vi "Tausand AB1000 Acquisition Example.vi"() -> ()   [LabVIEW 2015]
doc: "Example of a complete acquisition system using a Tausand Abacus.\n\nIncludes device identification, live settings changes and live data reading.\nData is shown in tables, graphs and saved in plain text files.\nUses a producer-consumer design pattern."
uses:
  <instrlib>/Tausand AB1000/Examples/sub vi/connectionState.ctl
  <instrlib>/Tausand AB1000/Public/Controls/settings4ch.ctl
  <instrlib>/Tausand AB1000/Public/Controls/configMultipleCoincRing.ctl
  <instrlib>/Tausand AB1000/Examples/sub vi/defaultSettings.ctl
  <instrlib>/Tausand AB1000/Public/Controls/deviceTypeRing.ctl
  <instrlib>/Tausand AB1000/Public/Controls/settings2ch.ctl
  <instrlib>/Tausand AB1000/Public/Controls/counters2ch.ctl
  <instrlib>/Tausand AB1000/Public/Controls/counters4ch.ctl
  <vilib>/Utility/miscctls.llb/LVRowAndColumnUnsignedTypeDef.ctl
  <instrlib>/Tausand AB1000/Public/Controls/channelRing.ctl
  <vilib>/Utility/file.llb/Write Delimited Spreadsheet (string).vi
  <vilib>/Utility/file.llb/Read Delimited Spreadsheet (string).vi
  <instrlib>/Tausand AB1000/Tausand AB1000.lvlib
panel:
  out "ref ctrls":T1
  out "timer-settings 2":timestamp
  in  "butLoadDefSett":bool
  out "ref indics":T2
  out "dafafile header":string[](array[string])
  in  "settings 2ch":T3={"sampling"=1000, "coincidence_window"=10, "delay_A"=0, "delay_B"=0, "sleep_A"=0, "sleep_B"=0} {"sleep_B" max=100 step=5; "sleep_A" max=100 step=5; "delay_B" max=100 step=5; "delay_A" max=100 step=5; "coincidence_window" min=5 max=50000 step=5; "sampling" items=["1ms"=1, "2ms"=2, "5ms"=5, "10ms"=10, "20ms"=20, "50ms"=50, "100ms"=100, "200ms"=200, "500ms"=500, "1s"=1000, "2s"=2000, "5s"=5000, "10s"=10000, "20s"=20000, "50s"=50000, "100s"=100000, "200s"=200000, "500s"=500000, "1000s"=1000000]}
  in  "settings 4ch":T4={"sampling"=1000, "coincidence_window"=10, "delay_A"=0, "delay_B"=0, "delay_C"=0, "delay_D"=0, "sleep_A"=0, "sleep_B"=0, "sleep_C"=0, "sleep_D"=0, "config_multiple_1"=240} {"config_multiple_1" items=["ABC"=224, "ABD"=208, "ACD"=176, "BCD"=112, "ABCD"=240]; "sleep_D" max=100 step=5; "sleep_C" max=100 step=5; "sleep_B" max=100 step=5; "sleep_A" max=100 step=5; "delay_D" max=100 step=5; "delay_C" max=100 step=5; "delay_B" max=100 step=5; "delay_A" max=100 step=5; "coincidence_window" min=5 max=10000 step=5; "sampling" items=["1ms"=1, "2ms"=2, "3ms"=3, "4ms"=4, "5ms"=5, "6ms"=6, "7ms"=7, "8ms"=8, "9ms"=9, "10ms"=10, "11ms"=11, "12ms"=12, "13ms"=13, "14ms"=14, "15ms"=15, "16ms"=16, "17ms"=17, "18ms"=18, "19ms"=19, "20ms"=20, "21ms"=21, "22ms"=22, "23ms"=23, "24ms"=24, "25ms"=25, "26ms"=26, "27ms"=27, "28ms"=28, "29ms"=29, "30ms"=30, "31ms"=31, "32ms"=32, "33ms"=33, "34ms"=34, "35ms"=35, "36ms"=36, "37ms"=37, "38ms"=38, "39ms"=39, "40ms"=40, "41ms"=41, "42ms"=42, "43ms"=43, "44ms"=44, "45ms"=45, "46ms"=46, "47ms"=47, "48ms"=48, "49ms"=49, "50ms"=50, "51ms"=51, "52ms"=52, "53ms"=53, "54ms"=54, "55ms"=55, "56ms"=56, "57ms"=57, "58ms"=58, "59ms"=59, "60ms"=60, "61ms"=61, "62ms"=62, "63ms"=63, "64ms"=64, "65ms"=65, "66ms"=66, "67ms"=67, "68ms"=68, "69ms"=69, "70ms"=70, "71ms"=71, "72ms"=72, "73ms"=73, "74ms"=74, "75ms"=75, "76ms"=76, "77ms"=77, "78ms"=78, "79ms"=79, "80ms"=80, "81ms"=81, "82ms"=82, "83ms"=83, "84ms"=84, "85ms"=85, "86ms"=86, "87ms"=87, "88ms"=88, "89ms"=89, "90ms"=90, "91ms"=91, "92ms"=92, "93ms"=93, "94ms"=94, "95ms"=95, "96ms"=96, "97ms"=97, "98ms"=98, "99ms"=99, "100ms"=100, "110ms"=110, "120ms"=120, "130ms"=130, "140ms"=140, "150ms"=150, "160ms"=160, "170ms"=170, "180ms"=180, "190ms"=190, "200ms"=200, "210ms"=210, "220ms"=220, "230ms"=230, "240ms"=240, "250ms"=250, "260ms"=260, "270ms"=270, "280ms"=280, "290ms"=290, "300ms"=300, "310ms"=310, "320ms"=320, "330ms"=330, "340ms"=340, "350ms"=350, "360ms"=360, "370ms"=370, "380ms"=380, "390ms"=390, "400ms"=400, "410ms"=410, "420ms"=420, "430ms"=430, "440ms"=440, "450ms"=450, "460ms"=460, "470ms"=470, "480ms"=480, "490ms"=490, "500ms"=500, "510ms"=510, "520ms"=520, "530ms"=530, "540ms"=540, "550ms"=550, "560ms"=560, "570ms"=570, "580ms"=580, "590ms"=590, "600ms"=600, "610ms"=610, "620ms"=620, "630ms"=630, "640ms"=640, "650ms"=650, "660ms"=660, "670ms"=670, "680ms"=680, "690ms"=690, "700ms"=700, "710ms"=710, "720ms"=720, "730ms"=730, "740ms"=740, "750ms"=750, "760ms"=760, "770ms"=770, "780ms"=780, "790ms"=790, "800ms"=800, "810ms"=810, "820ms"=820, "830ms"=830, "840ms"=840, "850ms"=850, "860ms"=860, "870ms"=870, "880ms"=880, "890ms"=890, "900ms"=900, "910ms"=910, "920ms"=920, "930ms"=930, "940ms"=940, "950ms"=950, "960ms"=960, "970ms"=970, "980ms"=980, "990ms"=990, "1,0s"=1000, "1,1s"=1100, "1,2s"=1200, "1,3s"=1300, "1,4s"=1400, "1,5s"=1500, "1,6s"=1600, "1,7s"=1700, "1,8s"=1800, "1,9s"=1900, "2,0s"=2000, "2,1s"=2100, "2,2s"=2200, "2,3s"=2300, "2,4s"=2400, "2,5s"=2500, "2,6s"=2600, "2,7s"=2700, "2,8s"=2800, "2,9s"=2900, "3,0s"=3000, "3,1s"=3100, "3,2s"=3200, "3,3s"=3300, "3,4s"=3400, "3,5s"=3500, "3,6s"=3600, "3,7s"=3700, "3,8s"=3800, "3,9s"=3900, "4,0s"=4000, "4,1s"=4100, "4,2s"=4200, "4,3s"=4300, "4,4s"=4400, "4,5s"=4500, "4,6s"=4600, "4,7s"=4700, "4,8s"=4800, "4,9s"=4900, "5,0s"=5000, "5,1s"=5100, "5,2s"=5200, "5,3s"=5300, "5,4s"=5400, "5,5s"=5500, "5,6s"=5600, "5,7s"=5700, "5,8s"=5800, "5,9s"=5900, "6,0s"=6000, "6,1s"=6100, "6,2s"=6200, "6,3s"=6300, "6,4s"=6400, "6,5s"=6500, "6,6s"=6600, "6,7s"=6700, "6,8s"=6800, "6,9s"=6900, "7,0s"=7000, "7,1s"=7100, "7,2s"=7200, "7,3s"=7300, "7,4s"=7400, "7,5s"=7500, "7,6s"=7600, "7,7s"=7700, "7,8s"=7800, "7,9s"=7900, "8,0s"=8000, "8,1s"=8100, "8,2s"=8200, "8,3s"=8300, "8,4s"=8400, "8,5s"=8500, "8,6s"=8600, "8,7s"=8700, "8,8s"=8800, "8,9s"=8900, "9,0s"=9000, "9,1s"=9100, "9,2s"=9200, "9,3s"=9300, "9,4s"=9400, "9,5s"=9500, "9,6s"=9600, "9,7s"=9700, "9,8s"=9800, "9,9s"=9900, "10s"=10000, "11s"=11000, "12s"=12000, "13s"=13000, "14s"=14000, "15s"=15000, "16s"=16000, "17s"=17000, "18s"=18000, "19s"=19000, "20s"=20000, "21s"=21000, "22s"=22000, "23s"=23000, "24s"=24000, "25s"=25000, "26s"=26000, "27s"=27000, "28s"=28000, "29s"=29000, "30s"=30000, "31s"=31000, "32s"=32000, "33s"=33000, "34s"=34000, "35s"=35000, "36s"=36000, "37s"=37000, "38s"=38000, "39s"=39000, "40s"=40000, "41s"=41000, "42s"=42000, "43s"=43000, "44s"=44000, "45s"=45000, "46s"=46000, "47s"=47000, "48s"=48000, "49s"=49000, "50s"=50000, "51s"=51000, "52s"=52000, "53s"=53000, "54s"=54000, "55s"=55000, "56s"=56000, "57s"=57000, "58s"=58000, "59s"=59000, "60s"=60000, "61s"=61000, "62s"=62000, "63s"=63000, "64s"=64000, "65s"=65000, "66s"=66000, "67s"=67000, "68s"=68000, "69s"=69000, "70s"=70000, "71s"=71000, "72s"=72000, "73s"=73000, "74s"=74000, "75s"=75000, "76s"=76000, "77s"=77000, "78s"=78000, "79s"=79000, "80s"=80000, "81s"=81000, "82s"=82000, "83s"=83000, "84s"=84000, "85s"=85000, "86s"=86000, "87s"=87000, "88s"=88000, "89s"=89000, "90s"=90000, "91s"=91000, "92s"=92000, "93s"=93000, "94s"=94000, "95s"=95000, "96s"=96000, "97s"=97000, "98s"=98000, "99s"=99000, "100s"=100000, "110s"=110000, "120s"=120000, "130s"=130000, "140s"=140000, "150s"=150000, "160s"=160000, "170s"=170000, "180s"=180000, "190s"=190000, "200s"=200000, "210s"=210000, "220s"=220000, "230s"=230000, "240s"=240000, "250s"=250000, "260s"=260000, "270s"=270000, "280s"=280000, "290s"=290000, "300s"=300000, "310s"=310000, "320s"=320000, "330s"=330000, "340s"=340000, "350s"=350000, "360s"=360000, "370s"=370000, "380s"=380000, "390s"=390000, "400s"=400000, "410s"=410000, "420s"=420000, "430s"=430000, "440s"=440000, "450s"=450000, "460s"=460000, "470s"=470000, "480s"=480000, "490s"=490000, "500s"=500000, "510s"=510000, "520s"=520000, "530s"=530000, "540s"=540000, "550s"=550000, "560s"=560000, "570s"=570000, "580s"=580000, "590s"=590000, "600s"=600000, "610s"=610000, "620s"=620000, "630s"=630000, "640s"=640000, "650s"=650000, "660s"=660000, "670s"=670000, "680s"=680000, "690s"=690000, "700s"=700000, "710s"=710000, "720s"=720000, "730s"=730000, "740s"=740000, "750s"=750000, "760s"=760000, "770s"=770000, "780s"=780000, "790s"=790000, "800s"=800000, "810s"=810000, "820s"=820000, "830s"=830000, "840s"=840000, "850s"=850000, "860s"=860000, "870s"=870000, "880s"=880000, "890s"=890000, "900s"=900000, "910s"=910000, "920s"=920000, "930s"=930000, "940s"=940000, "950s"=950000, "960s"=960000, "970s"=970000, "980s"=980000, "990s"=990000, "1000s"=1000000]}
  out "device type":T6 items=["any"=0, "AB1002"=1002, "AB1004"=1004, "AB1502"=1502, "AB1504"=1504, "AB2002"=2002, "AB2004"=2004, "AB2502"=2502, "AB2504"=2504]
  out "path-defsettings":path
  out "delimiter":string
  out "default settings":T7={"autogenerate"=FALSE, "datetime"=FALSE, "from_device"=FALSE, "directory"="", "file_prefix"="", "settings_suffix"="", "delimiter"="", "extension"="", "Abacus settings"={"sampling"=0, "coincidence_window"=0, "delay_A"=0, "delay_B"=0, "delay_C"=0, "delay_D"=0, "sleep_A"=0, "sleep_B"=0, "sleep_C"=0, "sleep_D"=0, "config_multiple_1"=240}} {"Abacus settings"."config_multiple_1" items=["ABC"=224, "ABD"=208, "ACD"=176, "BCD"=112, "ABCD"=240]; "Abacus settings"."sleep_D" max=100 step=5; "Abacus settings"."sleep_C" max=100 step=5; "Abacus settings"."sleep_B" max=100 step=5; "Abacus settings"."sleep_A" max=100 step=5; "Abacus settings"."delay_D" max=100 step=5; "Abacus settings"."delay_C" max=100 step=5; "Abacus settings"."delay_B" max=100 step=5; "Abacus settings"."delay_A" max=100 step=5; "Abacus settings"."coincidence_window" min=5 max=10000 step=5; "Abacus settings"."sampling" items=["1ms"=1, "2ms"=2, "3ms"=3, "4ms"=4, "5ms"=5, "6ms"=6, "7ms"=7, "8ms"=8, "9ms"=9, "10ms"=10, "11ms"=11, "12ms"=12, "13ms"=13, "14ms"=14, "15ms"=15, "16ms"=16, "17ms"=17, "18ms"=18, "19ms"=19, "20ms"=20, "21ms"=21, "22ms"=22, "23ms"=23, "24ms"=24, "25ms"=25, "26ms"=26, "27ms"=27, "28ms"=28, "29ms"=29, "30ms"=30, "31ms"=31, "32ms"=32, "33ms"=33, "34ms"=34, "35ms"=35, "36ms"=36, "37ms"=37, "38ms"=38, "39ms"=39, "40ms"=40, "41ms"=41, "42ms"=42, "43ms"=43, "44ms"=44, "45ms"=45, "46ms"=46, "47ms"=47, "48ms"=48, "49ms"=49, "50ms"=50, "51ms"=51, "52ms"=52, "53ms"=53, "54ms"=54, "55ms"=55, "56ms"=56, "57ms"=57, "58ms"=58, "59ms"=59, "60ms"=60, "61ms"=61, "62ms"=62, "63ms"=63, "64ms"=64, "65ms"=65, "66ms"=66, "67ms"=67, "68ms"=68, "69ms"=69, "70ms"=70, "71ms"=71, "72ms"=72, "73ms"=73, "74ms"=74, "75ms"=75, "76ms"=76, "77ms"=77, "78ms"=78, "79ms"=79, "80ms"=80, "81ms"=81, "82ms"=82, "83ms"=83, "84ms"=84, "85ms"=85, "86ms"=86, "87ms"=87, "88ms"=88, "89ms"=89, "90ms"=90, "91ms"=91, "92ms"=92, "93ms"=93, "94ms"=94, "95ms"=95, "96ms"=96, "97ms"=97, "98ms"=98, "99ms"=99, "100ms"=100, "110ms"=110, "120ms"=120, "130ms"=130, "140ms"=140, "150ms"=150, "160ms"=160, "170ms"=170, "180ms"=180, "190ms"=190, "200ms"=200, "210ms"=210, "220ms"=220, "230ms"=230, "240ms"=240, "250ms"=250, "260ms"=260, "270ms"=270, "280ms"=280, "290ms"=290, "300ms"=300, "310ms"=310, "320ms"=320, "330ms"=330, "340ms"=340, "350ms"=350, "360ms"=360, "370ms"=370, "380ms"=380, "390ms"=390, "400ms"=400, "410ms"=410, "420ms"=420, "430ms"=430, "440ms"=440, "450ms"=450, "460ms"=460, "470ms"=470, "480ms"=480, "490ms"=490, "500ms"=500, "510ms"=510, "520ms"=520, "530ms"=530, "540ms"=540, "550ms"=550, "560ms"=560, "570ms"=570, "580ms"=580, "590ms"=590, "600ms"=600, "610ms"=610, "620ms"=620, "630ms"=630, "640ms"=640, "650ms"=650, "660ms"=660, "670ms"=670, "680ms"=680, "690ms"=690, "700ms"=700, "710ms"=710, "720ms"=720, "730ms"=730, "740ms"=740, "750ms"=750, "760ms"=760, "770ms"=770, "780ms"=780, "790ms"=790, "800ms"=800, "810ms"=810, "820ms"=820, "830ms"=830, "840ms"=840, "850ms"=850, "860ms"=860, "870ms"=870, "880ms"=880, "890ms"=890, "900ms"=900, "910ms"=910, "920ms"=920, "930ms"=930, "940ms"=940, "950ms"=950, "960ms"=960, "970ms"=970, "980ms"=980, "990ms"=990, "1,0s"=1000, "1,1s"=1100, "1,2s"=1200, "1,3s"=1300, "1,4s"=1400, "1,5s"=1500, "1,6s"=1600, "1,7s"=1700, "1,8s"=1800, "1,9s"=1900, "2,0s"=2000, "2,1s"=2100, "2,2s"=2200, "2,3s"=2300, "2,4s"=2400, "2,5s"=2500, "2,6s"=2600, "2,7s"=2700, "2,8s"=2800, "2,9s"=2900, "3,0s"=3000, "3,1s"=3100, "3,2s"=3200, "3,3s"=3300, "3,4s"=3400, "3,5s"=3500, "3,6s"=3600, "3,7s"=3700, "3,8s"=3800, "3,9s"=3900, "4,0s"=4000, "4,1s"=4100, "4,2s"=4200, "4,3s"=4300, "4,4s"=4400, "4,5s"=4500, "4,6s"=4600, "4,7s"=4700, "4,8s"=4800, "4,9s"=4900, "5,0s"=5000, "5,1s"=5100, "5,2s"=5200, "5,3s"=5300, "5,4s"=5400, "5,5s"=5500, "5,6s"=5600, "5,7s"=5700, "5,8s"=5800, "5,9s"=5900, "6,0s"=6000, "6,1s"=6100, "6,2s"=6200, "6,3s"=6300, "6,4s"=6400, "6,5s"=6500, "6,6s"=6600, "6,7s"=6700, "6,8s"=6800, "6,9s"=6900, "7,0s"=7000, "7,1s"=7100, "7,2s"=7200, "7,3s"=7300, "7,4s"=7400, "7,5s"=7500, "7,6s"=7600, "7,7s"=7700, "7,8s"=7800, "7,9s"=7900, "8,0s"=8000, "8,1s"=8100, "8,2s"=8200, "8,3s"=8300, "8,4s"=8400, "8,5s"=8500, "8,6s"=8600, "8,7s"=8700, "8,8s"=8800, "8,9s"=8900, "9,0s"=9000, "9,1s"=9100, "9,2s"=9200, "9,3s"=9300, "9,4s"=9400, "9,5s"=9500, "9,6s"=9600, "9,7s"=9700, "9,8s"=9800, "9,9s"=9900, "10s"=10000, "11s"=11000, "12s"=12000, "13s"=13000, "14s"=14000, "15s"=15000, "16s"=16000, "17s"=17000, "18s"=18000, "19s"=19000, "20s"=20000, "21s"=21000, "22s"=22000, "23s"=23000, "24s"=24000, "25s"=25000, "26s"=26000, "27s"=27000, "28s"=28000, "29s"=29000, "30s"=30000, "31s"=31000, "32s"=32000, "33s"=33000, "34s"=34000, "35s"=35000, "36s"=36000, "37s"=37000, "38s"=38000, "39s"=39000, "40s"=40000, "41s"=41000, "42s"=42000, "43s"=43000, "44s"=44000, "45s"=45000, "46s"=46000, "47s"=47000, "48s"=48000, "49s"=49000, "50s"=50000, "51s"=51000, "52s"=52000, "53s"=53000, "54s"=54000, "55s"=55000, "56s"=56000, "57s"=57000, "58s"=58000, "59s"=59000, "60s"=60000, "61s"=61000, "62s"=62000, "63s"=63000, "64s"=64000, "65s"=65000, "66s"=66000, "67s"=67000, "68s"=68000, "69s"=69000, "70s"=70000, "71s"=71000, "72s"=72000, "73s"=73000, "74s"=74000, "75s"=75000, "76s"=76000, "77s"=77000, "78s"=78000, "79s"=79000, "80s"=80000, "81s"=81000, "82s"=82000, "83s"=83000, "84s"=84000, "85s"=85000, "86s"=86000, "87s"=87000, "88s"=88000, "89s"=89000, "90s"=90000, "91s"=91000, "92s"=92000, "93s"=93000, "94s"=94000, "95s"=95000, "96s"=96000, "97s"=97000, "98s"=98000, "99s"=99000, "100s"=100000, "110s"=110000, "120s"=120000, "130s"=130000, "140s"=140000, "150s"=150000, "160s"=160000, "170s"=170000, "180s"=180000, "190s"=190000, "200s"=200000, "210s"=210000, "220s"=220000, "230s"=230000, "240s"=240000, "250s"=250000, "260s"=260000, "270s"=270000, "280s"=280000, "290s"=290000, "300s"=300000, "310s"=310000, "320s"=320000, "330s"=330000, "340s"=340000, "350s"=350000, "360s"=360000, "370s"=370000, "380s"=380000, "390s"=390000, "400s"=400000, "410s"=410000, "420s"=420000, "430s"=430000, "440s"=440000, "450s"=450000, "460s"=460000, "470s"=470000, "480s"=480000, "490s"=490000, "500s"=500000, "510s"=510000, "520s"=520000, "530s"=530000, "540s"=540000, "550s"=550000, "560s"=560000, "570s"=570000, "580s"=580000, "590s"=590000, "600s"=600000, "610s"=610000, "620s"=620000, "630s"=630000, "640s"=640000, "650s"=650000, "660s"=660000, "670s"=670000, "680s"=680000, "690s"=690000, "700s"=700000, "710s"=710000, "720s"=720000, "730s"=730000, "740s"=740000, "750s"=750000, "760s"=760000, "770s"=770000, "780s"=780000, "790s"=790000, "800s"=800000, "810s"=810000, "820s"=820000, "830s"=830000, "840s"=840000, "850s"=850000, "860s"=860000, "870s"=870000, "880s"=880000, "890s"=890000, "900s"=900000, "910s"=910000, "920s"=920000, "930s"=930000, "940s"=940000, "950s"=950000, "960s"=960000, "970s"=970000, "980s"=980000, "990s"=990000, "1000s"=1000000]}
  out "settings_old":T4={"sampling"=1000, "coincidence_window"=10, "delay_A"=0, "delay_B"=0, "delay_C"=0, "delay_D"=0, "sleep_A"=0, "sleep_B"=0, "sleep_C"=0, "sleep_D"=0, "config_multiple_1"=0} {"config_multiple_1" items=["ABC"=224, "ABD"=208, "ACD"=176, "BCD"=112, "ABCD"=240]; "sleep_D" max=100 step=1; "sleep_C" max=100 step=1; "sleep_B" max=100 step=1; "sleep_A" max=100 step=1; "delay_D" max=100 step=1; "delay_C" max=100 step=1; "delay_B" max=100 step=1; "delay_A" max=100 step=1; "coincidence_window" min=1 max=10000 step=1; "sampling" items=["1ms"=1, "2ms"=2, "3ms"=3, "4ms"=4, "5ms"=5, "6ms"=6, "7ms"=7, "8ms"=8, "9ms"=9, "10ms"=10, "11ms"=11, "12ms"=12, "13ms"=13, "14ms"=14, "15ms"=15, "16ms"=16, "17ms"=17, "18ms"=18, "19ms"=19, "20ms"=20, "21ms"=21, "22ms"=22, "23ms"=23, "24ms"=24, "25ms"=25, "26ms"=26, "27ms"=27, "28ms"=28, "29ms"=29, "30ms"=30, "31ms"=31, "32ms"=32, "33ms"=33, "34ms"=34, "35ms"=35, "36ms"=36, "37ms"=37, "38ms"=38, "39ms"=39, "40ms"=40, "41ms"=41, "42ms"=42, "43ms"=43, "44ms"=44, "45ms"=45, "46ms"=46, "47ms"=47, "48ms"=48, "49ms"=49, "50ms"=50, "51ms"=51, "52ms"=52, "53ms"=53, "54ms"=54, "55ms"=55, "56ms"=56, "57ms"=57, "58ms"=58, "59ms"=59, "60ms"=60, "61ms"=61, "62ms"=62, "63ms"=63, "64ms"=64, "65ms"=65, "66ms"=66, "67ms"=67, "68ms"=68, "69ms"=69, "70ms"=70, "71ms"=71, "72ms"=72, "73ms"=73, "74ms"=74, "75ms"=75, "76ms"=76, "77ms"=77, "78ms"=78, "79ms"=79, "80ms"=80, "81ms"=81, "82ms"=82, "83ms"=83, "84ms"=84, "85ms"=85, "86ms"=86, "87ms"=87, "88ms"=88, "89ms"=89, "90ms"=90, "91ms"=91, "92ms"=92, "93ms"=93, "94ms"=94, "95ms"=95, "96ms"=96, "97ms"=97, "98ms"=98, "99ms"=99, "100ms"=100, "110ms"=110, "120ms"=120, "130ms"=130, "140ms"=140, "150ms"=150, "160ms"=160, "170ms"=170, "180ms"=180, "190ms"=190, "200ms"=200, "210ms"=210, "220ms"=220, "230ms"=230, "240ms"=240, "250ms"=250, "260ms"=260, "270ms"=270, "280ms"=280, "290ms"=290, "300ms"=300, "310ms"=310, "320ms"=320, "330ms"=330, "340ms"=340, "350ms"=350, "360ms"=360, "370ms"=370, "380ms"=380, "390ms"=390, "400ms"=400, "410ms"=410, "420ms"=420, "430ms"=430, "440ms"=440, "450ms"=450, "460ms"=460, "470ms"=470, "480ms"=480, "490ms"=490, "500ms"=500, "510ms"=510, "520ms"=520, "530ms"=530, "540ms"=540, "550ms"=550, "560ms"=560, "570ms"=570, "580ms"=580, "590ms"=590, "600ms"=600, "610ms"=610, "620ms"=620, "630ms"=630, "640ms"=640, "650ms"=650, "660ms"=660, "670ms"=670, "680ms"=680, "690ms"=690, "700ms"=700, "710ms"=710, "720ms"=720, "730ms"=730, "740ms"=740, "750ms"=750, "760ms"=760, "770ms"=770, "780ms"=780, "790ms"=790, "800ms"=800, "810ms"=810, "820ms"=820, "830ms"=830, "840ms"=840, "850ms"=850, "860ms"=860, "870ms"=870, "880ms"=880, "890ms"=890, "900ms"=900, "910ms"=910, "920ms"=920, "930ms"=930, "940ms"=940, "950ms"=950, "960ms"=960, "970ms"=970, "980ms"=980, "990ms"=990, "1,0s"=1000, "1,1s"=1100, "1,2s"=1200, "1,3s"=1300, "1,4s"=1400, "1,5s"=1500, "1,6s"=1600, "1,7s"=1700, "1,8s"=1800, "1,9s"=1900, "2,0s"=2000, "2,1s"=2100, "2,2s"=2200, "2,3s"=2300, "2,4s"=2400, "2,5s"=2500, "2,6s"=2600, "2,7s"=2700, "2,8s"=2800, "2,9s"=2900, "3,0s"=3000, "3,1s"=3100, "3,2s"=3200, "3,3s"=3300, "3,4s"=3400, "3,5s"=3500, "3,6s"=3600, "3,7s"=3700, "3,8s"=3800, "3,9s"=3900, "4,0s"=4000, "4,1s"=4100, "4,2s"=4200, "4,3s"=4300, "4,4s"=4400, "4,5s"=4500, "4,6s"=4600, "4,7s"=4700, "4,8s"=4800, "4,9s"=4900, "5,0s"=5000, "5,1s"=5100, "5,2s"=5200, "5,3s"=5300, "5,4s"=5400, "5,5s"=5500, "5,6s"=5600, "5,7s"=5700, "5,8s"=5800, "5,9s"=5900, "6,0s"=6000, "6,1s"=6100, "6,2s"=6200, "6,3s"=6300, "6,4s"=6400, "6,5s"=6500, "6,6s"=6600, "6,7s"=6700, "6,8s"=6800, "6,9s"=6900, "7,0s"=7000, "7,1s"=7100, "7,2s"=7200, "7,3s"=7300, "7,4s"=7400, "7,5s"=7500, "7,6s"=7600, "7,7s"=7700, "7,8s"=7800, "7,9s"=7900, "8,0s"=8000, "8,1s"=8100, "8,2s"=8200, "8,3s"=8300, "8,4s"=8400, "8,5s"=8500, "8,6s"=8600, "8,7s"=8700, "8,8s"=8800, "8,9s"=8900, "9,0s"=9000, "9,1s"=9100, "9,2s"=9200, "9,3s"=9300, "9,4s"=9400, "9,5s"=9500, "9,6s"=9600, "9,7s"=9700, "9,8s"=9800, "9,9s"=9900, "10s"=10000, "11s"=11000, "12s"=12000, "13s"=13000, "14s"=14000, "15s"=15000, "16s"=16000, "17s"=17000, "18s"=18000, "19s"=19000, "20s"=20000, "21s"=21000, "22s"=22000, "23s"=23000, "24s"=24000, "25s"=25000, "26s"=26000, "27s"=27000, "28s"=28000, "29s"=29000, "30s"=30000, "31s"=31000, "32s"=32000, "33s"=33000, "34s"=34000, "35s"=35000, "36s"=36000, "37s"=37000, "38s"=38000, "39s"=39000, "40s"=40000, "41s"=41000, "42s"=42000, "43s"=43000, "44s"=44000, "45s"=45000, "46s"=46000, "47s"=47000, "48s"=48000, "49s"=49000, "50s"=50000, "51s"=51000, "52s"=52000, "53s"=53000, "54s"=54000, "55s"=55000, "56s"=56000, "57s"=57000, "58s"=58000, "59s"=59000, "60s"=60000, "61s"=61000, "62s"=62000, "63s"=63000, "64s"=64000, "65s"=65000, "66s"=66000, "67s"=67000, "68s"=68000, "69s"=69000, "70s"=70000, "71s"=71000, "72s"=72000, "73s"=73000, "74s"=74000, "75s"=75000, "76s"=76000, "77s"=77000, "78s"=78000, "79s"=79000, "80s"=80000, "81s"=81000, "82s"=82000, "83s"=83000, "84s"=84000, "85s"=85000, "86s"=86000, "87s"=87000, "88s"=88000, "89s"=89000, "90s"=90000, "91s"=91000, "92s"=92000, "93s"=93000, "94s"=94000, "95s"=95000, "96s"=96000, "97s"=97000, "98s"=98000, "99s"=99000, "100s"=100000, "110s"=110000, "120s"=120000, "130s"=130000, "140s"=140000, "150s"=150000, "160s"=160000, "170s"=170000, "180s"=180000, "190s"=190000, "200s"=200000, "210s"=210000, "220s"=220000, "230s"=230000, "240s"=240000, "250s"=250000, "260s"=260000, "270s"=270000, "280s"=280000, "290s"=290000, "300s"=300000, "310s"=310000, "320s"=320000, "330s"=330000, "340s"=340000, "350s"=350000, "360s"=360000, "370s"=370000, "380s"=380000, "390s"=390000, "400s"=400000, "410s"=410000, "420s"=420000, "430s"=430000, "440s"=440000, "450s"=450000, "460s"=460000, "470s"=470000, "480s"=480000, "490s"=490000, "500s"=500000, "510s"=510000, "520s"=520000, "530s"=530000, "540s"=540000, "550s"=550000, "560s"=560000, "570s"=570000, "580s"=580000, "590s"=590000, "600s"=600000, "610s"=610000, "620s"=620000, "630s"=630000, "640s"=640000, "650s"=650000, "660s"=660000, "670s"=670000, "680s"=680000, "690s"=690000, "700s"=700000, "710s"=710000, "720s"=720000, "730s"=730000, "740s"=740000, "750s"=750000, "760s"=760000, "770s"=770000, "780s"=780000, "790s"=790000, "800s"=800000, "810s"=810000, "820s"=820000, "830s"=830000, "840s"=840000, "850s"=850000, "860s"=860000, "870s"=870000, "880s"=880000, "890s"=890000, "900s"=900000, "910s"=910000, "920s"=920000, "930s"=930000, "940s"=940000, "950s"=950000, "960s"=960000, "970s"=970000, "980s"=980000, "990s"=990000, "1000s"=1000000]}
  out "sttgs changed?":bool[](array[boolean])
  out "connection state":T8
  out "timer-reconnect":timestamp
  out "status":string
  out "path-new":path
  out "error":errorcluster
  out "path-settingsOld":path
  out "path-settings":path
  out "timer-settings":timestamp
  out "timer-readRequest":timestamp
  in  "Tab Control":T9(tab)
  out "dataTable":string[][](table)
  out "counters 2ch":T10
  out "counters 4ch":T11
  out "graph-A":cluster{timestamp[], u32[]}(graph) caption="small graph A"
  out "graph-B":cluster{timestamp[], u32[]}(graph) caption="small graph B"
  out "graph-C":cluster{timestamp[], u32[]}(graph) caption="small graph C"
  out "graph-D":cluster{timestamp[], u32[]}(graph) caption="small graph D"
  out "graph coinc":cluster{timestamp[], u32[]}[](graph)
  out "graph-A-S":cluster{timestamp[], u32[]}(graph) caption="small graph A"
  out "graph-B-S":cluster{timestamp[], u32[]}(graph) caption="small graph B"
  out "graph-C-S":cluster{timestamp[], u32[]}(graph) caption="small graph C"
  out "graph-D-S":cluster{timestamp[], u32[]}(graph) caption="small graph D"
  in  "butDisconnect":bool
  in  "butConnect":bool
  in  "butUnlockSett":bool
  in  "butStopAcq":bool
  in  "butStartAcq":bool
  out "path-fileOld":path
  in  "path-file":path caption="Save as"
  out "timer-begin":timestamp
  out "timer-nextRead":timestamp
  out "timer-lastRead":timestamp
  out "timer-current":timestamp
  out "abacus VISA":refnum<visa-resource-name>
  in  "butExit":bool
  # "Settings"
  # "January 2023"
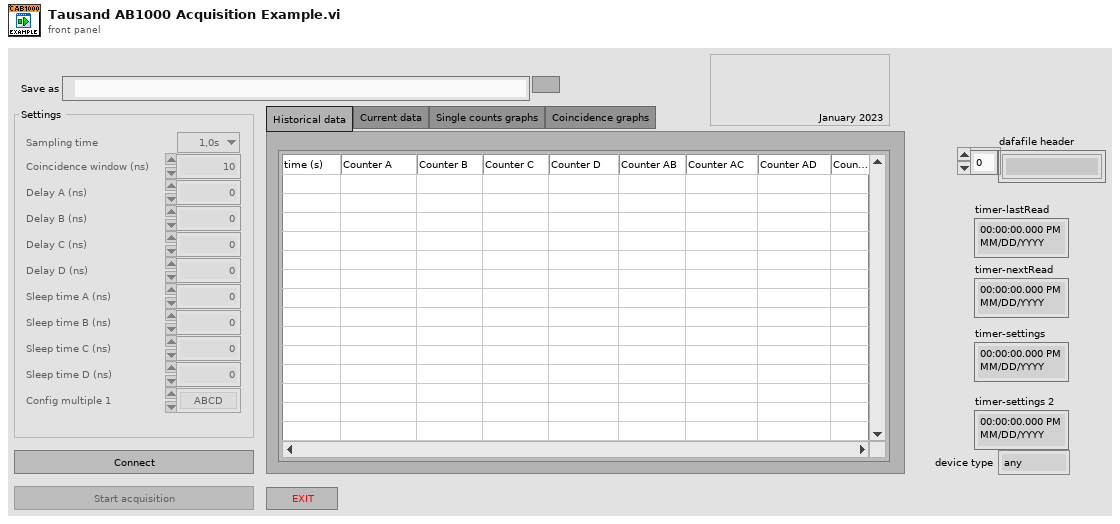
[diagram p1: front panel]
types:
  T1 = cluster{"butConnect":refnum<vi>, "butDisconnect":refnum<vi>, "butStartAcq":refnum<vi>, "butStopAcq":refnum<vi>, "butLoadDefSett":refnum<vi>, "butUnlockSett":refnum<vi>, "settings 2ch":refnum<vi>, "settings 4ch":refnum<vi>}
  T2 = cluster{"counters 2ch":refnum<vi>, "counters 4ch":refnum<vi>, "dataTable":refnum<vi>, "graph coinc":refnum<vi>, "graph-A":refnum<vi>, "graph-A-S":refnum<vi>, "graph-B":refnum<vi>, "graph-B-S":refnum<vi>, "graph-C":refnum<vi>, "graph-C-S":refnum<vi>, "graph-D":refnum<vi>, "graph-D-S":refnum<vi>}
  T3 = typedef "Tausand AB1000.lvlib/settings2ch.ctl" = cluster{"sampling":u32, "coincidence_window":u32, "delay_A":u32, "delay_B":u32, "sleep_A":u32, "sleep_B":u32}
  T4 = typedef "Tausand AB1000.lvlib/settings4ch.ctl" = cluster{"sampling":u32, "coincidence_window":u32, "delay_A":u32, "delay_B":u32, "delay_C":u32, "delay_D":u32, "sleep_A":u32, "sleep_B":u32, "sleep_C":u32, "sleep_D":u32, "config_multiple_1":T5}
  T5 = typedef "Tausand AB1000.lvlib/configMultipleCoincRing.ctl" = u16
  T6 = typedef "Tausand AB1000.lvlib/deviceTypeRing.ctl" = u16
  T7 = typedef "defaultSettings.ctl" = cluster{"autogenerate":bool, "datetime":bool, "from_device":bool, "directory":string, "file_prefix":string, "settings_suffix":string, "delimiter":string, "extension":string, "Abacus settings":T4}
  T8 = typedef "connectionState.ctl" = enum16{"disconnected", "connected", "acquiring data", "connection error", "acquisition error"}
  T9 = enum32{"Historical data", "Current data", "Single counts graphs", "Coincidence graphs"}
  T10 = typedef "Tausand AB1000.lvlib/counters2ch.ctl" = cluster{"counter_A":u32, "counter_B":u32, "counter_AB":u32, "counters_ID":u32, "time_left":u32}
  T11 = typedef "Tausand AB1000.lvlib/counters4ch.ctl" = cluster{"counter_A":u32, "counter_B":u32, "counter_C":u32, "counter_D":u32, "counter_AB":u32, "counter_AC":u32, "counter_AD":u32, "counter_BC":u32, "counter_BD":u32, "counter_CD":u32, "counter_multiple_1":u32, "counters_ID":u32, "time_left":u32}
  T12 = cluster{"seconds since 1Jan1904":timestamp, "counters 4ch":T11}[]
  T13 = typedef "Semaphore RefNum" = refnum<k1>
  T14 = cluster{"semaphore files":T13, "semaphore port":T13, "notifier read request":refnum<notifier>, "queue data":refnum<queue>, "queue instructions":refnum<queue>}
  T15 = cluster{"seconds since 1Jan1904":timestamp, "counters 4ch":T11}
  T16 = cluster{"sampling":bool, "coincidence_window":bool, "delay_A":bool, "delay_B":bool, "delay_C":bool, "delay_D":bool, "sleep_A":bool, "sleep_B":bool, "sleep_C":bool, "sleep_D":bool, "config_multiple_1":bool}
  T17 = enum8{"Enabled", "Disabled", "Disabled and Grayed Out"}
  T18 = cluster{"counter_A":u32, "counter_B":u32, "counter_C":u32, "counter_D":u32, "counter_AB":u32, "counter_AC":u32, "counter_AD":u32, "counter_BC":u32, "counter_BD":u32, "counter_CD":u32, "counter_multiple_1":u32, "counters_ID":u32, "time_left":u32}
  T19 = typedef "LVRowAndColumnUnsignedTypeDef.ctl" = cluster{"Row":u32, "Column":u32}
  T20 = cluster{"[0]":u32, "[1]":u32, "[2]":u32, "[3]":u32, "[4]":u32, "[5]":u32, "[6]":u32, "[7]":u32, "[8]":u32, "[9]":u32, "[10]":u32}
  T21 = typedef "abacus4ch.lvlib/settings4ch.ctl" = cluster{"sampling":u32, "coincidence_window":u32, "delay_A":u32, "delay_B":u32, "delay_C":u32, "delay_D":u32, "sleep_A":u32, "sleep_B":u32, "sleep_C":u32, "sleep_D":u32, "config_multiple_1":T22}
  T22 = typedef "abacus4ch.lvlib/configMultipleCoincRing.ctl" = u16
  T23 = typedef "Tausand AB1000.lvlib/channelRing.ctl" = u8
  T24 = cluster{"read time":timestamp, "output cluster 4ch":T11}
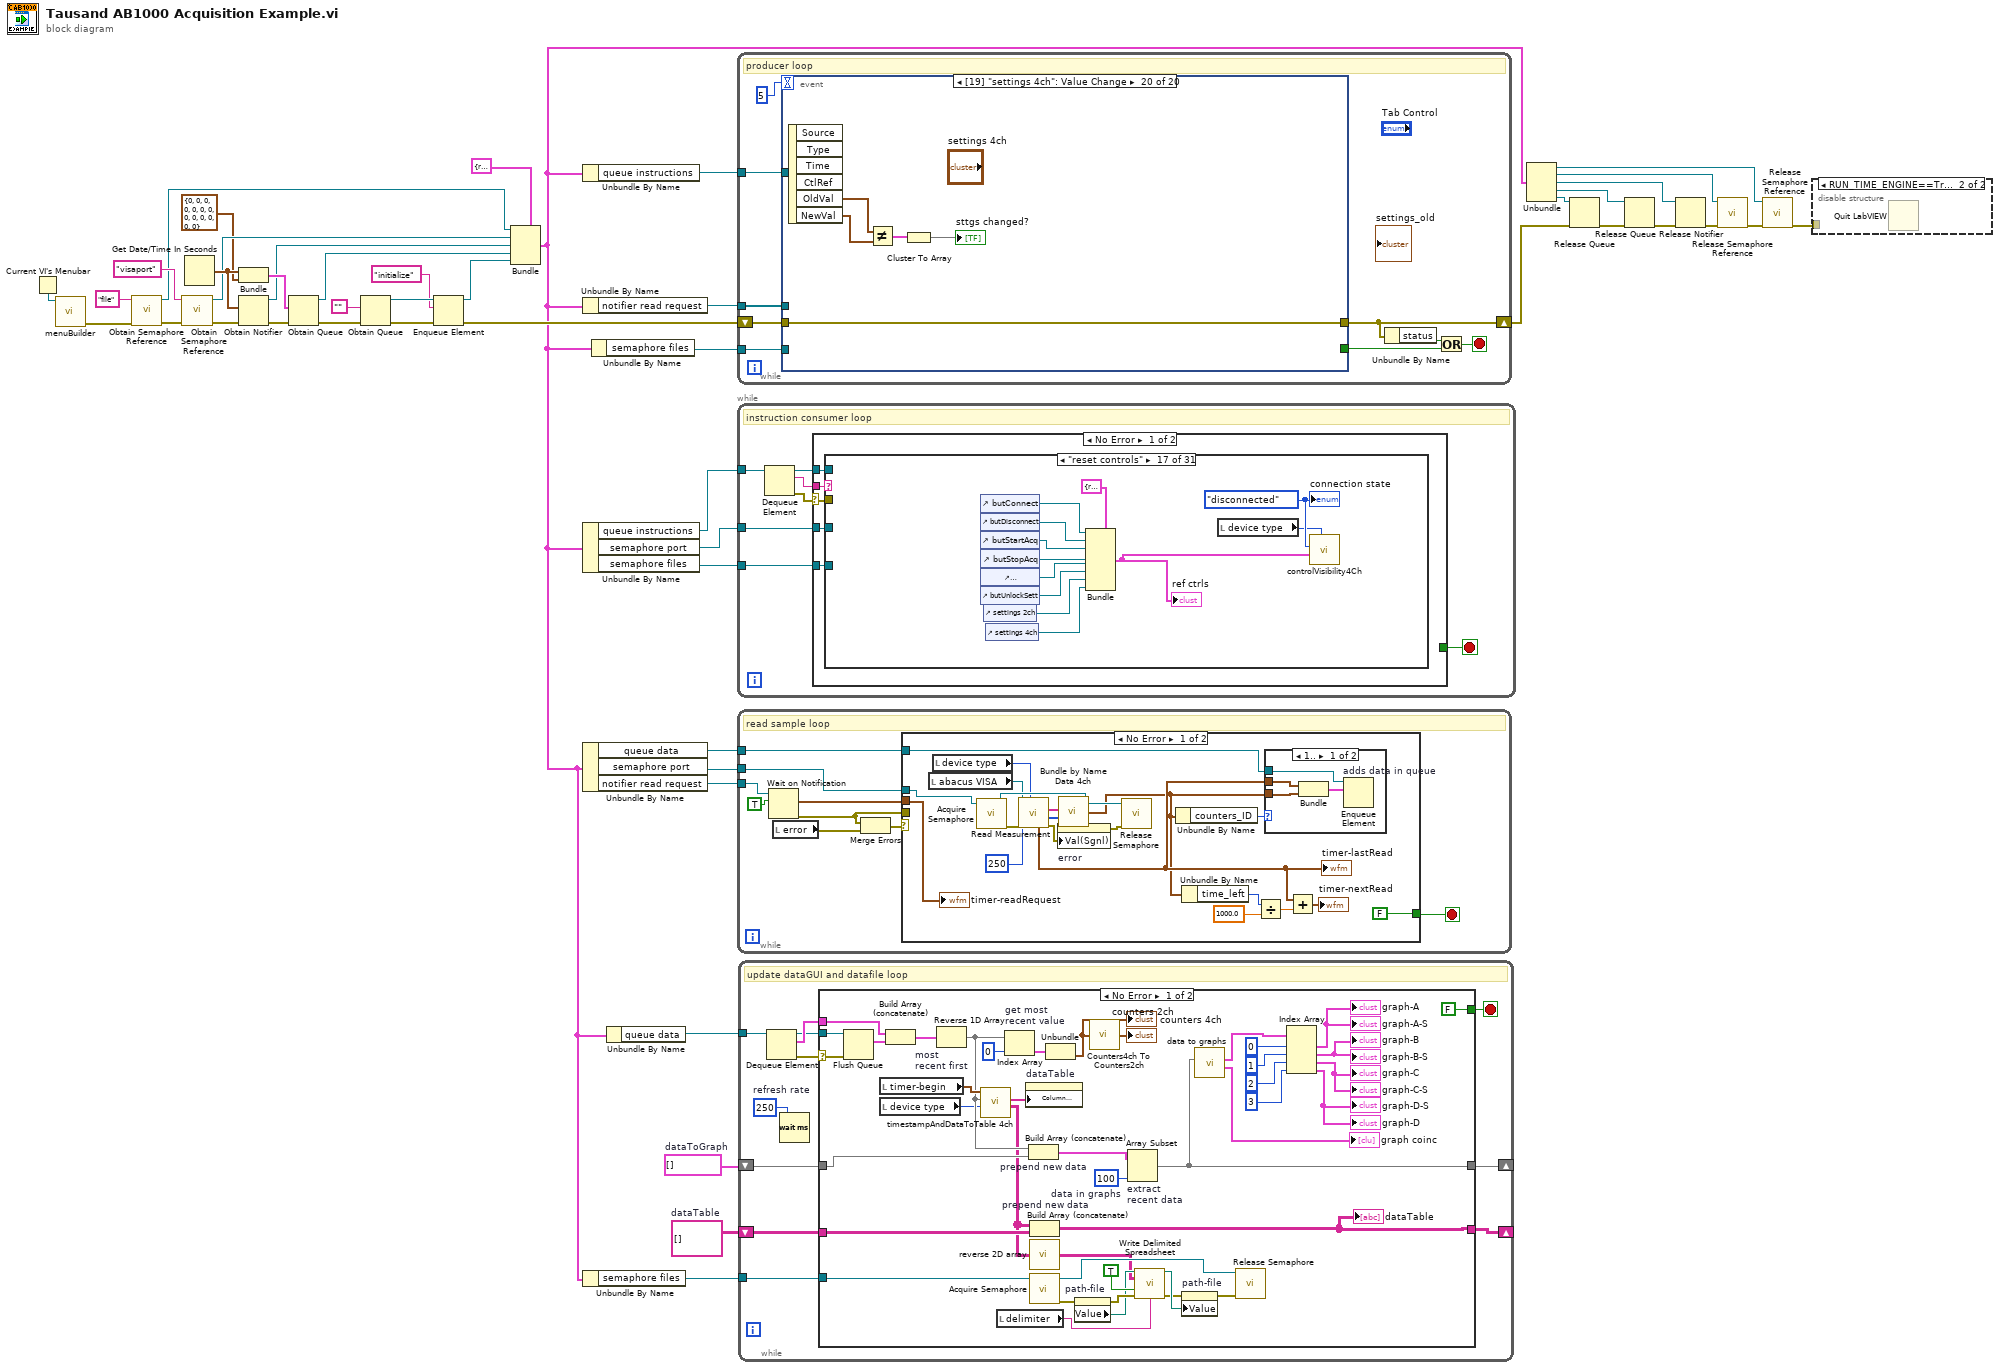
[diagram p0: block diagram]
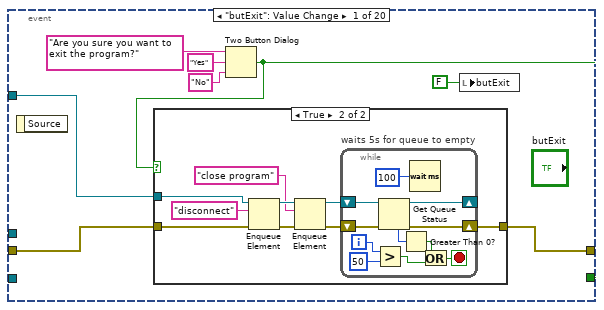
[diagram p2: hidden frame]
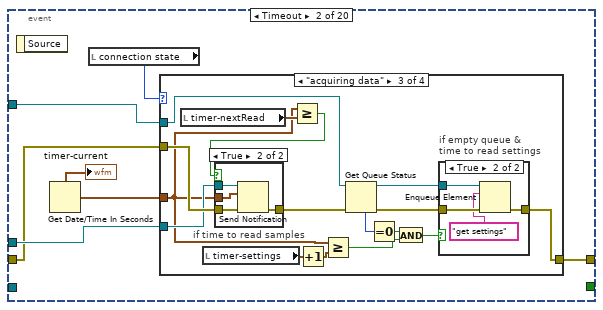
[diagram p4: hidden frame]
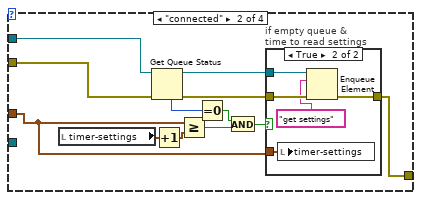
[diagram p6: hidden frame]
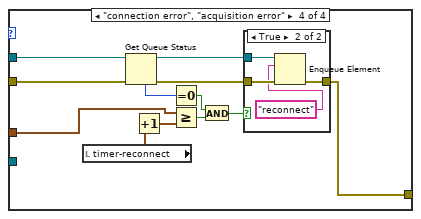
[diagram p10: hidden frame]
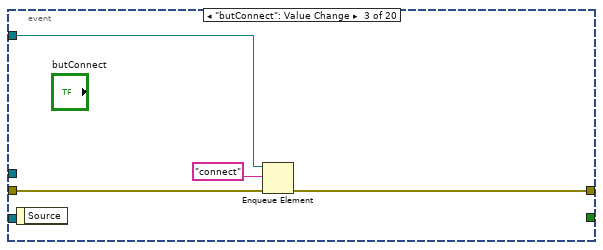
[diagram p12: hidden frame]
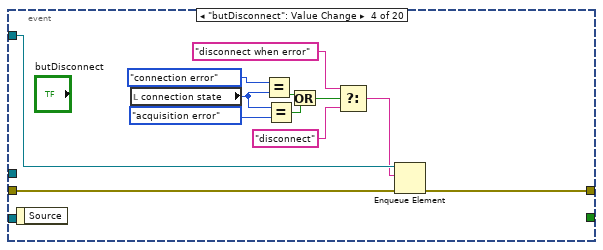
[diagram p13: hidden frame]
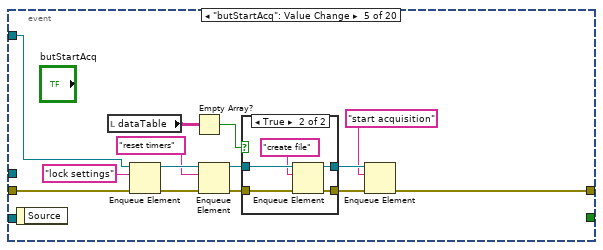
[diagram p14: hidden frame]
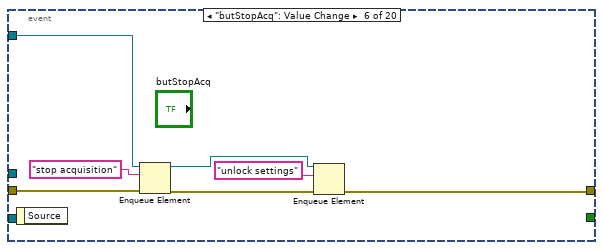
[diagram p16: hidden frame]
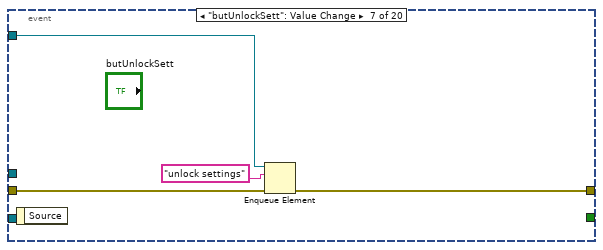
[diagram p17: hidden frame]
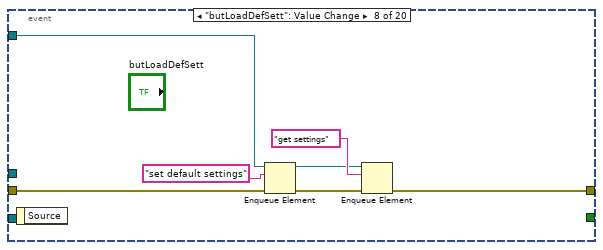
[diagram p18: hidden frame]
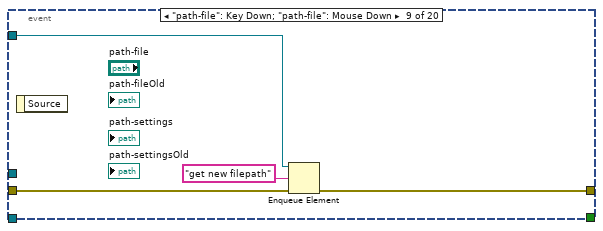
[diagram p19: hidden frame]
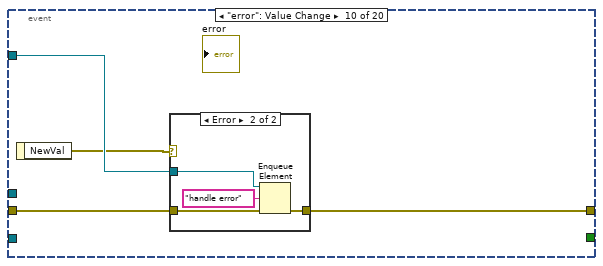
[diagram p20: hidden frame]
diagram:
  w1 = string[][] []  # dataTable
  w2 = T12 []  # dataToGraph
  n1 = Current VI's Menubar() -> (w7:refnum<k9>)
  n2 = call <instrlib>:"menuBuilder.vi"("Menu in"=w7) -> ("error out"=w8:errorcluster)  [unwired: 10 in]
  n3 = call <vilib>:"Obtain Semaphore Reference.vi"("error in (no error)"=w8, "name (unnamed)"="file") -> ("error out"=w34:errorcluster, "semaphore"=w13:T13)  [unwired: 3 in, 1 out]
  n4 = call <vilib>:"Obtain Semaphore Reference.vi"("error in (no error)"=w34, "name (unnamed)"="visaport") -> ("error out"=w37:errorcluster, "semaphore"=w32:T13)  [unwired: 3 in, 1 out]
  n5 = Get Date/Time In Seconds() -> (seconds since 1Jan1904=w36:timestamp)
  n6 = Bundle("seconds since 1Jan1904"=w36, "counters 4ch"=T11 {"counter_A"=0, "counter_B"=0, "counter_C"=0, "counter_D"=0, "counter_AB"=0, "counter_AC"=0, "counter_AD"=0, "counter_BC"=0, "counter_BD"=0, "counter_CD"=0, "counter_multiple_1"=0, "counters_ID"=0, "time_left"=0}) -> (w46:T15)  [unwired: 1 in]
  n7 = Obtain Notifier(notification data type=w36, error in (no error)=w37) -> (notifier out=w31:refnum<notifier>, error out=w45:errorcluster)  [unwired: 2 in, 1 out]
  n8 = Obtain Queue(element data type=w46, error in (no error)=w45) -> (queue out=w3:refnum<queue>, error out=w44:errorcluster)  [unwired: 3 in, 1 out]
  n9 = Obtain Queue(element data type="" ("str const"), error in (no error)=w44) -> (queue out=w40:refnum<queue>, error out=w42:errorcluster)  [unwired: 3 in, 1 out]
  n10 = Enqueue Element(queue=w40, element="initialize", error in (no error)=w42) -> (queue out=w30:refnum<queue>, error out=w41:errorcluster)  [unwired: 1 in, 1 out]
  n11 = Bundle(cluster=T14 {"semaphore files"=refnum, "semaphore port"=refnum, "notifier read request"=refnum, "queue data"=refnum, "queue instructions"=refnum}, "semaphore files"=w13, "semaphore port"=w32, "notifier read request"=w31, "queue data"=w3, "queue instructions"=w30) -> (w6:T14)
  n12 = Unbundle By Name(w6) -> ("queue instructions"=w9:refnum<queue>)
  n13 = Unbundle By Name(w6) -> ("notifier read request"=w11:refnum<notifier>)
  n14 = Unbundle By Name(w6) -> ("queue instructions"=w20:refnum<queue>, "semaphore port"=w19:T13, "semaphore files"=w18:T13)
  n15 = Unbundle By Name(w6) -> ("queue data"=w17:refnum<queue>, "semaphore port"=w16:T13, "notifier read request"=w15:refnum<notifier>)
  n16 = Unbundle By Name(w6) -> ("semaphore files"=w12:T13)
  n17 = Unbundle By Name(w6) -> ("semaphore files"=w5:T13)
  n18 = Unbundle By Name(w6) -> ("queue data"=w14:refnum<queue>)
  n19 = while {
    shift-right: [w53] -> w21
    shift-left: w41 -> [w56]
    tunnel: w11 -> [w50]
    tunnel: w9 -> [w49]
    tunnel: w5 -> [w48]
    stop <- w54 stop-if-true
    # "producer loop"
    n20 = event shown="[19] \"settings 4ch\": Value Change" {
      selector: _ -> [_ _ _ _ _ _ _ _ _ _ _ _ _ _ _ _ _ _ _ _]
      dyn-events: _ -> [_ _ _ _ _ _ _ _ _ _ _ _ _ _ _ _ _ _ _ _]
      timeout: 5 ("Numeric") -> [_ _ _ _ _ _ _ _ _ _ _ _ _ _ _ _ _ _ _ _]
      tunnel: w49 -> [w63 w90 w155 w167 w175 w195 w198 w206 w209 w216 _ w226 w259 w306 w310 w319 w327 w335 _ _]
      tunnel: w56 -> [w64 w89 w156 w169 w178 w196 w200 w207 w211 w214 w223 w228 w272 w304 w308 w312 w320 w328 w337 w344]
      tunnel: [w62 w88 w154 w168 w180 w192 w199 w204 w210 w215 w222 w227 w260 w305 w309 w318 w326 w334 w336 w344] -> w53
      tunnel: [w57 _ _ _ _ _ _ _ _ _ _ _ _ _ _ _ _ _ _ _] -> w55
      tunnel: w50 -> [_ w91 _ _ _ _ _ _ _ _ _ _ _ _ _ _ _ _ _ _]
      tunnel: w48 -> [_ _ _ _ _ _ _ _ _ _ _ _ w273 _ _ _ _ _ _ _]
      event "butExit": Value Change {
        n21 = event-data() -> ()  [unwired: 1 in, 1 out]
        n22 = Two Button Dialog(message="Are you sure you want to exit the program?", 1:"No" ("F button name (\"Cancel\")"), 2:"Yes" ("T button name (\"OK\")")) -> (T button?=w57:bool)
        n23 = case shown="True" w57 {
          tunnel: w64 -> [w65 w73]
          tunnel: w63 -> [_ w72]
          tunnel: [w65 w66] -> w62
          frame False {
          }
          frame True {
            n24 = Enqueue Element(queue=w72, element="disconnect", error in (no error)=w73) -> (queue out=w70:refnum<queue>, error out=w71:errorcluster)  [unwired: 1 in, 1 out]
            n25 = Enqueue Element(queue=w70, element="close program", error in (no error)=w71) -> (queue out=w67:refnum<queue>, error out=w68:errorcluster)  [unwired: 1 in, 1 out]
            n26 = while "waits 5s for queue to empty" {
              shift-right: [w83] -> w66
              shift-left: w68 -> [w85]
              shift-right: [w80] -> _
              shift-left: w67 -> [w84]
              i -> [w79]
              stop <- w75 stop-if-true
              n27 = Greater?(x=w79, y=50) -> (0:w76:bool)
              n28 = Get Queue Status(queue=w84, error in (no error)=w85) -> (queue out=w80:refnum<queue>, error out=w83:errorcluster, # elements in queue=w82:i32)  [unwired: 1 in, 5 out]
              n29 = Greater Than 0?(x=w82) -> (x > 0?=w77:bool)
              n30 = Wait (ms)(milliseconds to wait=u32 100 ("refresh rate")) -> ()  [unwired: 1 out]
              n31 = Or(x=w77, y=w76) -> (x .or. y?=w75:bool)
            }
          }
        }
        n32 = local write "butExit"(FALSE ("butStop")) -> ()
      }
      event Timeout {
        n33 = event-data() -> ()  [unwired: 1 in, 1 out]
        n34 = Get Date/Time In Seconds() -> (seconds since 1Jan1904=w87:timestamp)
        "timer-current" <- w87
        n35 = local read "connection state"() -> (w86:T8)
        n36 = case shown="\"acquiring data\"" w86 {
          tunnel: w89 -> [w92 w94 w114 w140]
          tunnel: w90 -> [_ w95 w117 w139]
          tunnel: [w92 w96 w118 w138] -> w88
          tunnel: w87 -> [_ w93 w111 w137]
          tunnel: w91 -> [_ _ w112 _]
          frame "disconnected", Default {
          }
          frame "connected" {
            n37 = local read "timer-settings"() -> (w99:timestamp)
            n38 = Get Queue Status(queue=w95, error in (no error)=w94) -> (queue out=w103:refnum<queue>, error out=w104:errorcluster, # elements in queue=w101:i32)  [unwired: 1 in, 5 out]
            n39 = Increment(x=w99) -> (x+1=w100:timestamp)
            n40 = Greater Or Equal?(x=w93, y=w100) -> (x >= y?=w97:bool)
            n41 = Equal To 0?(x=w101) -> (x = 0?=w98:bool)
            n42 = And(x=w98, y=w97) -> (x .and. y?=w102:bool)
            n43 = case "if empty queue &\ntime to read settings" shown="True" w102 {
              tunnel: w104 -> [w105 w110]
              tunnel: [w105 w109] -> w96
              tunnel: w103 -> [_ w108]
              tunnel: w93 -> [_ w106]
              frame False {
              }
              frame True {
                n44 = local write "timer-settings"(w106) -> ()
                n45 = Enqueue Element(queue=w108, element="get settings", error in (no error)=w110) -> (error out=w109:errorcluster)  [unwired: 1 in, 2 out]
              }
            }
          }
          frame "acquiring data" {
            n46 = local read "timer-nextRead"() -> (w116:timestamp)
            n47 = local read "timer-settings"() -> (w121:timestamp)
            n48 = Greater Or Equal?(x=w111, y=w116) -> (x >= y?=w115:bool)
            n49 = case "if time to read samples" shown="True" w115 {
              tunnel: [w127 w131] -> w113
              tunnel: w114 -> [w127 w130]
              tunnel: w112 -> [_ w129]
              tunnel: w111 -> [_ w128]
              frame False {
              }
              frame True {
                n50 = Send Notification(notification=w128, notifier=w129, error in (no error)=w130) -> (error out=w131:errorcluster)  [unwired: 1 out]
              }
            }
            n51 = Increment(x=w121) -> (x+1=w122:timestamp)
            n52 = Greater Or Equal?(x=w111, y=w122) -> (x >= y?=w119:bool)
            n53 = Get Queue Status(queue=w117, error in (no error)=w113) -> (queue out=w125:refnum<queue>, error out=w126:errorcluster, # elements in queue=w123:i32)  [unwired: 1 in, 5 out]
            n54 = Equal To 0?(x=w123) -> (x = 0?=w120:bool)
            n55 = And(x=w120, y=w119) -> (x .and. y?=w124:bool)
            n56 = case "if empty queue &\ntime to read settings" shown="True" w124 {
              tunnel: w126 -> [w132 w136]
              tunnel: [w132 w135] -> w118
              tunnel: w125 -> [_ w134]
              frame False {
              }
              frame True {
                n57 = Enqueue Element(queue=w134, element="get settings", error in (no error)=w136) -> (error out=w135:errorcluster)  [unwired: 1 in, 2 out]
              }
            }
          }
          frame "connection error", "acquisition error" {
            n58 = local read "timer-reconnect"() -> (w146:timestamp)
            n59 = Get Queue Status(queue=w139, error in (no error)=w140) -> (queue out=w142:refnum<queue>, error out=w141:errorcluster, # elements in queue=w144:i32)  [unwired: 1 in, 5 out]
            n60 = Increment(x=w146) -> (x+1=w145:timestamp)
            n61 = Equal To 0?(x=w144) -> (x = 0?=w147:bool)
            n62 = Greater Or Equal?(x=w137, y=w145) -> (x >= y?=w148:bool)
            n63 = And(x=w147, y=w148) -> (x .and. y?=w143:bool)
            n64 = case "if empty queue & time to try reconnection" shown="True" w143 {
              tunnel: w141 -> [w149 w153]
              tunnel: [w149 w152] -> w138
              tunnel: w142 -> [_ w151]
              frame False {
              }
              frame True {
                n65 = Enqueue Element(queue=w151, element="reconnect", error in (no error)=w153) -> (error out=w152:errorcluster)  [unwired: 1 in, 2 out]
              }
            }
          }
        }
      }
      event "butConnect": Value Change {
        n66 = event-data() -> ()  [unwired: 1 in, 1 out]
        n67 = Enqueue Element(queue=w155, element="connect", error in (no error)=w156) -> (error out=w154:errorcluster)  [unwired: 1 in, 2 out]
      }
      event "butDisconnect": Value Change {
        n68 = event-data() -> ()  [unwired: 1 in, 1 out]
        n69 = local read "connection state"() -> (w165:T8)
        n70 = Equal?(x=connectionState."connection error" ("connection state"), y=w165) -> (x = y?=w162:bool)
        n71 = Equal?(x=w165, y=connectionState."acquisition error" ("connection state")) -> (x = y?=w163:bool)
        n72 = Or(x=w162, y=w163) -> (x .or. y?=w161:bool)
        n73 = Select(t="disconnect when error" ("element"), s=w161, f="disconnect" ("element")) -> (s? t:f=w158:string)
        n74 = Enqueue Element(queue=w167, element=w158, error in (no error)=w169) -> (error out=w168:errorcluster)  [unwired: 1 in, 2 out]
      }
      event "butStartAcq": Value Change {
        n75 = event-data() -> ()  [unwired: 1 in, 1 out]
        n76 = local read "dataTable"() -> (w171:string[][])
        n77 = Enqueue Element(queue=w175, element="lock settings", error in (no error)=w178) -> (queue out=w174:refnum<queue>, error out=w177:errorcluster)  [unwired: 1 in, 1 out]
        n78 = Empty Array?(array=w171) -> (empty?=w170:bool)
        n79 = Enqueue Element(queue=w174, element="reset timers", error in (no error)=w177) -> (queue out=w182:refnum<queue>, error out=w183:errorcluster)  [unwired: 1 in, 1 out]
        n80 = case shown="True" w170 {
          tunnel: w183 -> [w185 w190]
          tunnel: w182 -> [w184 w189]
          tunnel: [w185 w188] -> w181
          tunnel: [w184 w187] -> w179
          frame False {
          }
          frame True {
            n81 = Enqueue Element(queue=w189, element="create file", error in (no error)=w190) -> (queue out=w187:refnum<queue>, error out=w188:errorcluster)  [unwired: 1 in, 1 out]
          }
        }
        n82 = Enqueue Element(queue=w179, element="start acquisition", error in (no error)=w181) -> (error out=w180:errorcluster)  [unwired: 1 in, 2 out]
      }
      event "butStopAcq": Value Change {
        n83 = event-data() -> ()  [unwired: 1 in, 1 out]
        n84 = Enqueue Element(queue=w195, element="stop acquisition", error in (no error)=w196) -> (queue out=w191:refnum<queue>, error out=w193:errorcluster)  [unwired: 1 in, 1 out]
        n85 = Enqueue Element(queue=w191, element="unlock settings", error in (no error)=w193) -> (error out=w192:errorcluster)  [unwired: 1 in, 2 out]
      }
      event "butUnlockSett": Value Change {
        n86 = event-data() -> ()  [unwired: 1 in, 1 out]
        n87 = Enqueue Element(queue=w198, element="unlock settings", error in (no error)=w200) -> (error out=w199:errorcluster)  [unwired: 1 in, 2 out]
      }
      event "butLoadDefSett": Value Change {
        n88 = event-data() -> ()  [unwired: 1 in, 1 out]
        n89 = Enqueue Element(queue=w206, element="set default settings", error in (no error)=w207) -> (queue out=w202:refnum<queue>, error out=w205:errorcluster)  [unwired: 1 in, 1 out]
        n90 = Enqueue Element(queue=w202, element="get settings", error in (no error)=w205) -> (error out=w204:errorcluster)  [unwired: 1 in, 2 out]
      }
      event "path-file": Key Down; "path-file": Mouse Down {
        n91 = event-data() -> ()  [unwired: 1 in, 1 out]
        n92 = Enqueue Element(queue=w209, element="get new filepath", error in (no error)=w211) -> (error out=w210:errorcluster)  [unwired: 1 in, 2 out]
      }
      event "error": Value Change {
        n93 = event-data() -> ("NewVal"=w213:errorcluster)  [unwired: 1 in]
        n94 = case shown="Error" w213 {
          tunnel: w214 -> [w217 w220]
          tunnel: w216 -> [_ w219]
          tunnel: [w217 w218] -> w215
          frame No Error {
          }
          frame Error {
            n95 = Enqueue Element(queue=w219, element="handle error", error in (no error)=w220) -> (error out=w218:errorcluster)  [unwired: 1 in, 2 out]
          }
        }
      }
      event Panel Close? {
        n96 = event-data() -> ()  [unwired: 1 in, 4 out]
        n97 = property on="butExit" class="Bool (strict)"(error in=w223, "Val(Sgnl)"=TRUE ("Value (Signaling)")) -> (error out=w222:errorcluster)  [unwired: 1 in, 1 out]
        n98 = event-data("Discard?"=TRUE) -> ()  [unwired: 1 in, 1 out]
      }
      event Menu Selection (User) {
        n99 = event-data() -> ("ItemTag"=w229:string)  [unwired: 1 in]
        n100 = case shown="\"About\"" w229 {
          tunnel: w228 -> [w230 w232 w237 w248 w250]
          tunnel: [w230 w231 w236 w247 w249] -> w227
          tunnel: w226 -> [_ _ _ w245 _]
          frame Default {
          }
          frame "Exit" {
            n101 = property on="butExit" class="Bool (strict)"(error in=w232, "Val(Sgnl)"=TRUE ("Value (Signaling)")) -> (error out=w231:errorcluster)  [unwired: 1 in, 1 out]
          }
          frame "Default settings" {
            w242 = 128  # call and forget
            n102 = vi-ref <instrlib>:"defaultSettingsDialog.vi"() -> (w241:refnum<vi>)
            n103 = local read "path-defsettings"() -> (w235:path)
            n104 = property class="VI"(reference=w241, error in=w237) -> (error out=w244:errorcluster, "Name"=w243:string)  [unwired: 1 out]
            n105 = control-ref of="default settings"() -> (w234:refnum<vi>)
            n106 = Open VI Reference(type specifier VI Refnum (for type only)=refnum<vi> refnum, vi path=w243, options=w242, error in (no error)=w244) -> (vi reference=w239:refnum<vi>, error out=w238:errorcluster)  [unwired: 2 in]
            n107 = call-by-ref "Start Asynchronous Call"(reference=w239, error in=w238, "default settings ref"=w234, "default settings path"=w235) -> (error out=w236:errorcluster)  [unwired: 9 in, 2 out]
          }
          frame "Save as" {
            n108 = Enqueue Element(queue=w245, element="get new filepath", error in (no error)=w248) -> (error out=w247:errorcluster)  [unwired: 1 in, 2 out]
          }
          frame "About" {
            w255 = 128  # call and forget
            n109 = vi-ref <instrlib>:"aboutDialog.vi"() -> (w254:refnum<vi>)
            n110 = property class="VI"(reference=w254, error in=w250) -> (error out=w257:errorcluster, "Name"=w256:string)  [unwired: 1 out]
            n111 = Open VI Reference(type specifier VI Refnum (for type only)=refnum<vi> refnum, vi path=w256, options=w255, error in (no error)=w257) -> (vi reference=w252:refnum<vi>, error out=w251:errorcluster)  [unwired: 2 in]
            n112 = call-by-ref "Start Asynchronous Call"(reference=w252, error in=w251) -> (error out=w249:errorcluster)  [unwired: 11 in, 2 out]
          }
        }
      }
      event Value Change {
        n113 = event-data() -> ("OldVal"=w266:T7, "NewVal"=w264:T7)  [unwired: 1 in]
        n114 = local read "path-settings"() -> (w281:path)
        n115 = local read "path-file"() -> (w275:path)
        n116 = call <instrlib>:"buildDefaultPath.vi"("default settings"=w264) -> ("settings path"=w282:path, "data path"=w271:path)  [unwired: 3 in]
        n117 = call <vilib>:"Acquire Semaphore.vi"("error in (no error)"=w272, "semaphore"=w273) -> ("error out"=w276:errorcluster, "semaphore out"=w278:T13)  [unwired: 3 in, 1 out]
        n118 = Not Equal?(x=w275, y=w271) -> (x != y?=w280:bool)
        n119 = Not Equal?(x=w282, y=w281) -> (x != y?=w279:bool)
        n120 = Or(x=w280, y=w279) -> (x .or. y?=w274:bool)
        n121 = case "path changed?" shown="True" w274 {
          tunnel: w259 -> [w296 w302]
          tunnel: w276 -> [w297 w301]
          tunnel: w271 -> [_ w299]
          tunnel: [w297 w300] -> w277
          tunnel: [w296 w298] -> w258
          frame False {
          }
          frame True {
            n122 = local write "path-new"(w299) -> ()
            n123 = Enqueue Element(queue=w302, element="rename files", error in (no error)=w301) -> (queue out=w298:refnum<queue>, error out=w300:errorcluster)  [unwired: 1 in, 1 out]
          }
        }
        n124 = Unbundle By Name(w266) -> ("delimiter"=w268:string)
        n125 = Unbundle By Name(w264) -> ("delimiter"=w267:string)
        n126 = Unbundle By Name(w266) -> ("Abacus settings"=w265:T4)
        n127 = Unbundle By Name(w264) -> ("Abacus settings"=w263:T4)
        n128 = Not Equal?(x=w268, y=w267) -> (x != y?=w270:bool)
        n129 = call <vilib>:"Release Semaphore.vi"("error in (no error)"=w277, "semaphore"=w278) -> ("error out"=w269:errorcluster)  [unwired: 4 in, 1 out]
        n130 = case "delimiter changed?" shown="True" w270 {
          tunnel: [w290 w294] -> w261
          tunnel: w258 -> [w289 w293]
          tunnel: w269 -> [w290 w292]
          tunnel: [w289 w291] -> w262
          frame False {
          }
          frame True {
            n131 = Enqueue Element(queue=w293, element="edit file delimiter", error in (no error)=w292) -> (queue out=w291:refnum<queue>, error out=w294:errorcluster)  [unwired: 1 in, 1 out]
          }
        }
        n132 = Not Equal?(x=w265, y=w263) -> (x != y?=w283:bool)
        n133 = case "def. settings changed?" shown="True" w283 {
          tunnel: w262 -> [_ w287]
          tunnel: w261 -> [w284 w286]
          tunnel: [w284 w285] -> w260
          frame False {
          }
          frame True {
            n134 = Enqueue Element(queue=w287, element="set default settings", error in (no error)=w286) -> (error out=w285:errorcluster)  [unwired: 1 in, 2 out]
          }
        }
      }
      event Value Change {
        n135 = event-data() -> ()  [unwired: 1 in, 2 out]
        n136 = Enqueue Element(queue=w306, element="set sampling", error in (no error)=w304) -> (error out=w305:errorcluster)  [unwired: 1 in, 2 out]
      }
      event Value Change {
        n137 = event-data() -> ()  [unwired: 1 in, 2 out]
        n138 = Enqueue Element(queue=w310, element="set coincidence window", error in (no error)=w308) -> (error out=w309:errorcluster)  [unwired: 1 in, 2 out]
      }
      event Value Change {
        n139 = event-data() -> ("CtlRef"=w317:refnum<vi>)  [unwired: 1 in, 2 out]
        n140 = property class="DigNum (strict)"(reference=w317) -> ("Label.Text"=w314:string)  [unwired: 1 in, 2 out]
        n141 = call <instrlib>:"getLastChar.vi"("string"=w314) -> ("last char"=w313:string)
        n142 = Concatenate Strings("set delay " ("element"), w313) -> (w315:string)
        n143 = Enqueue Element(queue=w319, element=w315, error in (no error)=w312) -> (error out=w318:errorcluster)  [unwired: 1 in, 2 out]
      }
      event Value Change {
        n144 = event-data() -> ("CtlRef"=w325:refnum<vi>)  [unwired: 1 in, 2 out]
        n145 = property class="DigNum (strict)"(reference=w325) -> ("Label.Text"=w322:string)  [unwired: 1 in, 2 out]
        n146 = call <instrlib>:"getLastChar.vi"("string"=w322) -> ("last char"=w321:string)
        n147 = Concatenate Strings("set sleep " ("element"), w321) -> (w323:string)
        n148 = Enqueue Element(queue=w327, element=w323, error in (no error)=w320) -> (error out=w326:errorcluster)  [unwired: 1 in, 2 out]
      }
      event Value Change {
        n149 = event-data() -> ("CtlRef"=w330:refnum<vi>)  [unwired: 1 in, 2 out]
        n150 = property class="Ring (strict)"(reference=w330) -> ("Label.Text"=w332:string)  [unwired: 1 in, 2 out]
        n151 = call <instrlib>:"getLastChar.vi"("string"=w332) -> ("last char"=w331:string)
        n152 = Concatenate Strings("set multi " ("element"), w331) -> (w329:string)
        n153 = Enqueue Element(queue=w335, element=w329, error in (no error)=w328) -> (error out=w334:errorcluster)  [unwired: 1 in, 2 out]
      }
      event Value Change {
        n154 = event-data() -> ()  [unwired: 1 in, 6 out]
        n155 = call <instrlib>:"Settings2ch To Settings4ch.vi"("settings2ch"="settings 2ch") -> ("settings4ch"=w338:T4)
        n156 = property on="settings 4ch" class="Clust (strict)"(error in=w337, "Val(Sgnl)"=w338) -> (error out=w336:errorcluster)  [unwired: 1 in, 1 out]
      }
      event Value Change {
        n157 = event-data() -> ("OldVal"=w343:T4, "NewVal"=w342:T4)  [unwired: 1 in, 4 out]
        n158 = Not Equal?(x=w343, y=w342) -> (x != y?=w341:T16)
        n159 = Cluster To Array(cluster=w341) -> (array=→"sttgs changed?":bool[])
      }
    }
    n160 = Unbundle By Name(w53) -> ("status"=w52:bool)
    n161 = Or(x=w52, y=w55) -> (x .or. y?=w54:bool)
  }
  n162 = while {
    tunnel: w20 -> [w345]
    tunnel: w19 -> [w348]
    tunnel: w18 -> [w347]
    stop <- w349 stop-if-true
    # "instruction consumer loop"
    n163 = Dequeue Element(queue=w345) -> (queue out=w346:refnum<queue>, element=w350:string, error out=w351:errorcluster)  [unwired: 2 in, 1 out]
    n164 = case shown="No Error" w351 {
      selector: w351 -> [w352 _]
      tunnel: w350 -> [w356 _]
      tunnel: [_ TRUE] -> w349
      tunnel: w348 -> [w355 _]
      tunnel: w347 -> [w354 _]
      tunnel: w346 -> [w353 _]
      frame No Error {
        n165 = case shown="\"reset controls\"" w356 {
          selector: w356 -> [_ _ _ _ _ _ _ _ _ _ _ _ _ _ _ _ _ _ _ _ _ _ w911 w966 _ _ w1046 _ _ _ _]
          tunnel: w355 -> [_ w372 _ _ w452 _ _ w497 _ w562 _ _ _ w664 w697 _ _ _ _ _ w845 w855 w910 w967 w1007 _ w1045 _ _ _ _]
          tunnel: w354 -> [w361 w371 w418 w422 w443 _ w474 w496 w540 w561 w598 _ _ _ w681 w746 _ _ _ _ w837 w854 w901 w957 w999 _ w1036 w1087 w1106 _ _]
          tunnel: w353 -> [_ w368 _ _ _ _ _ _ w547 _ w617 w651 _ w662 w692 _ _ _ _ _ _ _ _ _ _ w1018 _ _ _ _ _]
          tunnel: w352 -> [_ _ _ _ _ _ _ w495 w539 w560 w615 w650 _ _ _ _ _ _ _ _ _ w856 _ _ _ w1017 _ _ _ _ _]
          frame "close program" {
            n166 = local read "dataTable"() -> (w360:string[][])
            n167 = Empty Array?(array=w360) -> (empty?=w359:bool)
            n168 = case shown="True" w359 {
              tunnel: w361 -> [_ w367]
              frame False {
              }
              frame True {
                # "if no data taken, delete settings file"
                n169 = call <vilib>:"Acquire Semaphore.vi"("semaphore"=w367) -> ("error out"=w365:errorcluster, "semaphore out"=w366:T13)  [unwired: 4 in, 1 out]
                n170 = property on="path-settings" class="Path"(error in=w365) -> (error out=w363:errorcluster, "Value"=w364:path)  [unwired: 1 in, 1 out]
                n171 = Delete(path (use dialog)=w364, error in=w363) -> (error out=w362:errorcluster)  [unwired: 3 in, 2 out]
                n172 = call <vilib>:"Release Semaphore.vi"("error in (no error)"=w362, "semaphore"=w366) -> ()  [unwired: 4 in, 2 out]
              }
            }
            n173 = call <instrlib>:"prependTimestamp.vi"("string in"="Closing program" ("status str")) -> ("string out"=w357:string)  [unwired: 14 in]
            n174 = local write "status"(w357) -> ()
          }
          frame "connect" {
            n175 = call <instrlib>:"connectToDevice.vi"() -> ("selected device type"=w370:T6, "selected VISA"=w369:refnum<visa-resource-name>, "Cancelled?"=w374:bool)  [unwired: 8 in, 1 out]
            "device type" <- w370
            n176 = Not(x=w374) -> (.not. x?=w373:bool)
            n177 = case shown="True" w373 {
              tunnel: w372 -> [_ w380]
              tunnel: w371 -> [_ w379]
              tunnel: w370 -> [_ w378]
              tunnel: w369 -> [_ w377]
              tunnel: w368 -> [_ w376]
              frame False {
                n178 = local write "connection state"(connectionState."disconnected" ("connection state")) -> ()
              }
              frame True {
                n179 = stacked-sequence {
                  tunnel: w380 -> [w383 _ _]
                  tunnel: w379 -> [_ w394 _]
                  tunnel: w378 -> [_ w391 w402]
                  tunnel: w377 -> [w382 w392 _]
                  tunnel: w376 -> [w381 _ _]
                  frame #0 {
                    n180 = call <vilib>:"Acquire Semaphore.vi"("semaphore"=w383) -> ("error out"=w385:errorcluster, "semaphore out"=w386:T13)  [unwired: 4 in, 1 out]
                    n181 = call <instrlib>:"Open.vi"("error in (no error)"=w385, "VISA resource name"=w382) -> ("error out"=w384:errorcluster, "VISA resource name out"=→"abacus VISA":refnum<visa-resource-name>)  [unwired: 8 in]
                    n182 = call <vilib>:"Release Semaphore.vi"("error in (no error)"=w384, "semaphore"=w386) -> ("error out"=w388:errorcluster)  [unwired: 4 in, 1 out]
                    n183 = Enqueue Element(queue=w381, element="get initial settings", error in (no error)=w388) -> ()  [unwired: 1 in, 3 out]
                  }
                  frame #1 {
                    n184 = call <instrlib>:"connectionStatusString.vi"("connected? [T]"=TRUE, "device type"=w391, "Abacus VISA"=w392) -> ("String"=w393:string)  [unwired: 8 in]
                    n185 = call <vilib>:"Acquire Semaphore.vi"("semaphore"=w394) -> ("error out"=w398:errorcluster, "semaphore out"=w396:T13)  [unwired: 4 in, 1 out]
                    n186 = local read "delimiter"() -> (w400:string)
                    n187 = property on="path-settings" class="Path"(error in=w398) -> (error out=w399:errorcluster, "Value"=w397:path)  [unwired: 1 in, 1 out]
                    n188 = call <instrlib>:"writeSettingsFile4ch.vi"("delimiter (,)"=w400, "message (overrides settings)"=w393, "error in (no error)"=w399, "path"=w397) -> ("error out"=w401:errorcluster)  [unwired: 6 in, 1 out]
                    n189 = call <instrlib>:"prependTimestamp.vi"("string in"=w393) -> ("string out"=w395:string)  [unwired: 14 in]
                    n190 = call <vilib>:"Release Semaphore.vi"("error in (no error)"=w401, "semaphore"=w396) -> ()  [unwired: 4 in, 2 out]
                    n191 = local write "status"(w395) -> ()
                  }
                  frame #2 {
                    w403 = connectionState."connected" ("connection state")
                    n192 = local read "ref indics"() -> (w405:T2)
                    n193 = local read "ref ctrls"() -> (w404:T1)
                    n194 = local write "connection state"(w403) -> ()
                    n195 = call <instrlib>:"controlVisibility4Ch.vi"("device type [AB1004]"=w402, "ref controls"=w404, "connection state"=w403) -> ()  [unwired: 9 in]
                    n196 = call <instrlib>:"indicatorVisibility4Ch.vi"("device type [AB1004]"=w402, "ref indics"=w405) -> ()  [unwired: 10 in]
                  }
                }
              }
            }
          }
          frame "create file" {
            # "Clears the file if it exists, creates it if is new."
            n197 = local read "device type"() -> (w407:T6)
            n198 = call <instrlib>:"Get Channels From Device Type.vi"("device type"=w407) -> ("channels"=w406:i32)  [unwired: 4 in]
            n199 = case shown="2" w406 {
              tunnel: [string[] ["Time (s)", "Data ID", "Counts A", "Counts B", "Counts C", "Counts D", "Coincidences AB", "Coincidences AC", "Coincidences AD", "Coincidences BC", "Coincidences BD", "Coincidences CD", "Multi-fold"] string[] ["Time (s)", "Data ID", "Counts A", "Counts B", "Coincidences AB"]] -> w408
              frame 4, Default {
              }
              frame 2 {
              }
            }
            "dafafile header" <- w408
            n200 = call <vilib>:"Acquire Semaphore.vi"("semaphore"=w418) -> ("error out"=w412:errorcluster, "semaphore out"=w417:T13)  [unwired: 4 in, 1 out]
            n201 = local read "delimiter"() -> (w409:string)
            n202 = property on="path-file" class="Path"(error in=w412) -> (error out=w411:errorcluster, "Value"=w410:path)  [unwired: 1 in, 1 out]
            n203 = call-poly <vilib>:"Write Delimited Spreadsheet.vi"("file path (dialog if empty)"=w410, "1D data"=w408, "append to file? (F)"=FALSE, "error in (no error)"=w411, "delimiter (\\t)"=w409) -> ("new file path (Not A Path if cancelled)"=w415:path, "error out"=w414:errorcluster)  [unwired: 9 in]
            n204 = property on="path-file" class="Path"(error in=w414, "Value"=w415) -> (error out=w413:errorcluster)  [unwired: 1 in, 1 out]
            n205 = call <vilib>:"Release Semaphore.vi"("error in (no error)"=w413, "semaphore"=w417) -> ()  [unwired: 4 in, 2 out]
          }
          frame "create settings file" {
            n206 = local read "timer-begin"() -> (w429:timestamp)
            n207 = Format Date/Time String(time format string (%c)="%Y/%m/%d %H:%M:%S", seconds (now)=w429) -> (date/time string=w427:string)  [unwired: 1 in]
            n208 = call <vilib>:"Space Constant.vi"() -> ("String"=w430:string)
            n209 = Concatenate Strings("##### SETTINGS FILE #####\nTausand Abacus session began at", w430, w427) -> (w434:string)
            n210 = call <vilib>:"Acquire Semaphore.vi"("semaphore"=w422) -> ("error out"=w426:errorcluster, "semaphore out"=w425:T13)  [unwired: 4 in, 1 out]
            n211 = Build Array(w434) -> (w433:string[])
            n212 = property on="path-settings" class="Path"(error in=w426) -> (error out=w423:errorcluster, "Value"=w424:path)  [unwired: 1 in, 1 out]
            n213 = call-poly <vilib>:"Write Delimited Spreadsheet.vi"("file path (dialog if empty)"=w424, "1D data"=w433, "append to file? (F)"=FALSE, "error in (no error)"=w423) -> ("error out"=w421:errorcluster)  [unwired: 10 in, 1 out]
            n214 = call <vilib>:"Release Semaphore.vi"("error in (no error)"=w421, "semaphore"=w425) -> ()  [unwired: 4 in, 2 out]
          }
          frame "disconnect" {
            n215 = local read "abacus VISA"() -> (w437:refnum<visa-resource-name>)
            n216 = call <vilib>:"Acquire Semaphore.vi"("semaphore"=w452) -> ("error out"=w447:errorcluster, "semaphore out"=w448:T13)  [unwired: 4 in, 1 out]
            n217 = local read "device type"() -> (w436:T6)
            n218 = call <instrlib>:"Close.vi"("error in (no error)"=w447, "VISA resource name"=w437) -> ("error out"=w446:errorcluster)  [unwired: 9 in]
            n219 = call <vilib>:"Release Semaphore.vi"("error in (no error)"=w446, "semaphore"=w448) -> ()  [unwired: 4 in, 2 out]
            n220 = call <instrlib>:"connectionStatusString.vi"("connected? [T]"=FALSE, "device type"=w436, "Abacus VISA"=w437) -> ("String"=w438:string)  [unwired: 8 in]
            n221 = call <vilib>:"Acquire Semaphore.vi"("semaphore"=w443) -> ("error out"=w445:errorcluster, "semaphore out"=w444:T13)  [unwired: 4 in, 1 out]
            n222 = local read "delimiter"() -> (w439:string)
            n223 = property on="path-settings" class="Path"(error in=w445) -> (error out=w442:errorcluster, "Value"=w440:path)  [unwired: 1 in, 1 out]
            n224 = local read "connection state"() -> (w449:T8)
            n225 = call <instrlib>:"writeSettingsFile4ch.vi"("delimiter (,)"=w439, "message (overrides settings)"=w438, "error in (no error)"=w442, "path"=w440) -> ("error out"=w441:errorcluster)  [unwired: 6 in, 1 out]
            n226 = call <vilib>:"Release Semaphore.vi"("error in (no error)"=w441, "semaphore"=w444) -> ()  [unwired: 4 in, 2 out]
            n227 = case shown="\"connected\", Default" w449 {
              selector: w449 -> [_ w456 w457]
              tunnel: [connectionState."disconnected" ("connection state") w456 w457] -> w451
              tunnel: w438 -> [w453 _ _]
              frame "connected", Default {
                n228 = call <instrlib>:"prependTimestamp.vi"("string in"=w453) -> ("string out"=w454:string)  [unwired: 14 in]
                n229 = local write "status"(w454) -> ()
              }
              frame "connection error" {
              }
              frame "acquisition error" {
              }
            }
            n230 = local read "ref ctrls"() -> (w450:T1)
            n231 = local write "connection state"(w451) -> ()
            n232 = call <instrlib>:"controlVisibility4Ch.vi"("device type [AB1004]"=w436, "ref controls"=w450, "connection state"=w451) -> ()  [unwired: 9 in]
          }
          frame "disconnect when error" {
            w461 = connectionState."disconnected" ("connection state")
            n233 = local read "device type"() -> (w458:T6)
            n234 = local read "ref ctrls"() -> (w460:T1)
            n235 = property on="status" class="Str"("Text.TextColor"=u32 0) -> ()  [unwired: 2 in, 2 out]
            n236 = local write "connection state"(w461) -> ()
            n237 = call <instrlib>:"controlVisibility4Ch.vi"("device type [AB1004]"=w458, "ref controls"=w460, "connection state"=w461) -> ()  [unwired: 9 in]
          }
          frame "edit file delimiter" {
            n238 = call <vilib>:"Acquire Semaphore.vi"("semaphore"=w474) -> ("error out"=w470:errorcluster, "semaphore out"=w472:T13)  [unwired: 4 in, 1 out]
            n239 = local read "path-settings"() -> (w468:path)
            n240 = local read "default settings"() -> (w473:T7)
            n241 = local read "path-file"() -> (w469:path)
            n242 = property on="delimiter" class="Str"(error in=w470) -> (error out=w464:errorcluster, "Value"=w471:string)  [unwired: 1 in, 1 out]
            n243 = Build Array(w469, w468) -> (w467:path[])
            n244 = Unbundle By Name(w473) -> ("delimiter"=w463:string)
            n245 = case shown="\",\", \";\", Default" w463 {
              selector: w463 -> [_ _ w477]
              tunnel: [w475 "\t" w477] -> w462
              frame "Space", "space" {
                n246 = call <vilib>:"Space Constant.vi"() -> ("String"=w475:string)
              }
              frame "Tab", "tab" {
              }
              frame ",", ";", Default {
              }
            }
            n247 = for {
              tunnel: w471 -> [w483]
              tunnel: w462 -> [w482]
              shift-right: [w480] -> w466
              shift-left: w464 -> [w481]
              tunnel: w467 -> [w479] mode=indexing
              n248 = call <vilib>:"Is Path and Not Empty.vi"("path"=w479) -> ("Is Path and Not Empty?"=w484:bool)  [unwired: 4 in]
              n249 = call <vilib>:"Check if File or Folder Exists.vi"("path"=w479) -> ("file or folder exists?"=w485:bool)  [unwired: 8 in, 2 out]
              n250 = And(x=w484, y=w485) -> (x .and. y?=w478:bool)
              n251 = case shown="True" w478 {
                tunnel: w483 -> [_ w494]
                tunnel: w482 -> [_ w493]
                tunnel: w481 -> [w486 w489]
                tunnel: [w486 w488] -> w480
                tunnel: w479 -> [_ w487]
                frame False {
                }
                frame True {
                  n252 = call-poly <vilib>:"Read Delimited Spreadsheet.vi"("file path (dialog if empty)"=w487, "error in (no error)"=w489, "delimiter (\\t)"=w494) -> ("new file path (Not A Path if cancelled)"=w491:path, "all rows"=w492:string[][], "error out"=w490:errorcluster)  [unwired: 7 in, 3 out]
                  n253 = call-poly <vilib>:"Write Delimited Spreadsheet.vi"("file path (dialog if empty)"=w491, "2D data"=w492, "error in (no error)"=w490, "delimiter (\\t)"=w493) -> ("error out"=w488:errorcluster)  [unwired: 10 in, 1 out]
                }
              }
            }
            n254 = property on="delimiter" class="Str"(error in=w466, "Value"=w462) -> (error out=w465:errorcluster)  [unwired: 1 in, 1 out]
            n255 = call <vilib>:"Release Semaphore.vi"("error in (no error)"=w465, "semaphore"=w472) -> ()  [unwired: 4 in, 2 out]
          }
          frame "get initial settings" {
            n256 = local read "connection state"() -> (w498:T8)
            n257 = case shown="\"connected\"" w498 {
              tunnel: w497 -> [_ w505]
              tunnel: w496 -> [_ w504]
              tunnel: w495 -> [_ w503]
              frame "disconnected", Default {
              }
              frame "connected" {
                # "fake old values to\nforce file writing"
                n258 = local read "abacus VISA"() -> (w508:refnum<visa-resource-name>)
                n259 = local read "device type"() -> (w514:T6)
                n260 = call <vilib>:"Acquire Semaphore.vi"("error in (no error)"=w503, "semaphore"=w505) -> ("error out"=w511:errorcluster, "semaphore out"=w506:T13)  [unwired: 3 in, 1 out]
                n261 = Initialize Array(u32 99999 ("delay_C"), 11 ("dimension size")) -> (w502:u32[])
                n262 = call <instrlib>:"Query All Settings.vi"("device type"=w514, "error in (no error)"=w511, "read timeout (500 ms)"=u32 250 ("read timeout (10000 ms)"), "VISA Refnum in"=w508) -> ("error out"=w509:errorcluster, "values"=w516:u32[], "labels"=w515:string[], "checksum ok?"=w512:bool)  [unwired: 3 in, 1 out]
                n263 = Array To Cluster(array=w502) -> (cluster=w499:T20)
                n264 = case shown="True" w512 {
                  tunnel: w499 -> [_ w531]
                  tunnel: w509 -> [w517 w519]
                  tunnel: [w517 w520] -> w510
                  tunnel: w515 -> [_ w533]
                  tunnel: w516 -> [_ w532]
                  tunnel: w504 -> [_ w518]
                  frame False {
                  }
                  frame True {
                    n265 = local read "settings 4ch"() -> (w521:T4)
                    n266 = local read "delimiter"() -> (w526:string)
                    n267 = call <instrlib>:"Bundle by Name Settings 4ch.vi"("input cluster settings 4ch"=w521, "names"=w533, "values"=w532) -> ("output cluster settings 4ch"=w522:T4)  [unwired: 12 in]
                    n268 = call <vilib>:"Acquire Semaphore.vi"("error in (no error)"=w519, "semaphore"=w518) -> ("error out"=w530:errorcluster, "semaphore out"=w524:T13)  [unwired: 3 in, 1 out]
                    n269 = property on="path-settings" class="Path"(error in=w530) -> (error out=w529:errorcluster, "Value"=w527:path)  [unwired: 1 in, 1 out]
                    n270 = call <instrlib>:"Settings4ch To Settings2ch.vi"("settings4ch"=w522) -> ("settings2ch"=w523:T3)
                    n271 = Get Date/Time In Seconds() -> (seconds since 1Jan1904=w525:timestamp)
                    "timer-settings 2" <- w525
                    n272 = local write "settings 2ch"(w523) -> ()
                    n273 = local write "settings_old"(w522) -> ()
                    n274 = local write "settings 4ch"(w522) -> ()
                    n275 = call <instrlib>:"writeSettingsFile4ch.vi"("delimiter (,)"=w526, "timestamp (current)"=w525, "error in (no error)"=w529, "old settings"=w531, "new settings"=w522, "path"=w527) -> ("error out"=w528:errorcluster)  [unwired: 4 in, 1 out]
                    n276 = call <vilib>:"Release Semaphore.vi"("error in (no error)"=w528, "semaphore"=w524) -> ("error out"=w520:errorcluster)  [unwired: 4 in, 1 out]
                  }
                }
                n277 = property on="error" class="Clust (strict)"("Val(Sgnl)"=w510) -> (error out=w507:errorcluster)  [unwired: 2 in, 1 out]
                n278 = call <vilib>:"Release Semaphore.vi"("error in (no error)"=w507, "semaphore"=w506) -> ()  [unwired: 4 in, 2 out]
              }
            }
          }
          frame "get new filepath" {
            n279 = local read "default settings"() -> (w536:T7)
            n280 = Unbundle By Name(w536) -> ("extension"=w537:string)
            n281 = local read "path-file"() -> (w544:path)
            n282 = case shown="\".csv\"" w537 {
              selector: w537 -> [_ w552]
              tunnel: ["Plain text data file" ("pattern label") "CSV (comma dellimited)" ("pattern label")] -> w535
              tunnel: [".dat" ("pattern (all files)") w552] -> w534
              frame ".dat", Default {
              }
              frame ".csv" {
              }
            }
            n283 = Strip Path(path=w544) -> (name=w548:string)  [unwired: 1 out]
            n284 = call "File Dialog"("start path"=w544, "prompt"="Save as... ", "default name"=w548, "error in"=w539, "pattern (all files)"=w534, "pattern label"=w535) -> ("selected path"=w545:path, "cancelled"=w546:bool, "error out"=w538:errorcluster)  [unwired: 6 in, 1 out]
            n285 = call <vilib>:"Acquire Semaphore.vi"("error in (no error)"=w538, "semaphore"=w540) -> ("error out"=w543:errorcluster, "semaphore out"=w541:T13)  [unwired: 3 in, 1 out]
            n286 = case shown="False" w546 {
              tunnel: w547 -> [w557 _]
              tunnel: w543 -> [w556 w559]
              tunnel: w545 -> [w554 _]
              tunnel: [w555 w559] -> w542
              frame False {
                n287 = Enqueue Element(queue=w557, element="rename files", error in (no error)=w556) -> (error out=w555:errorcluster)  [unwired: 1 in, 2 out]
                "path-new" <- w554
              }
              frame True {
              }
            }
            n288 = call <vilib>:"Release Semaphore.vi"("error in (no error)"=w542, "semaphore"=w541) -> ()  [unwired: 4 in, 2 out]
          }
          frame "get settings" {
            n289 = local read "connection state"() -> (w563:T8)
            n290 = case shown="\"connected\", \"acquiring data\"" w563 {
              tunnel: w562 -> [_ w566]
              tunnel: w561 -> [_ w565]
              tunnel: w560 -> [_ w564]
              frame "disconnected", Default {
              }
              frame "connected", "acquiring data" {
                n291 = local read "abacus VISA"() -> (w569:refnum<visa-resource-name>)
                n292 = local read "device type"() -> (w577:T6)
                n293 = property on="settings 4ch" class="Clust (strict)"(error in=w564) -> (error out=w575:errorcluster, "Value"=w576:T4)  [unwired: 1 in, 1 out]
                n294 = call <vilib>:"Acquire Semaphore.vi"("error in (no error)"=w575, "semaphore"=w566) -> ("error out"=w572:errorcluster, "semaphore out"=w567:T13)  [unwired: 3 in, 1 out]
                n295 = call <instrlib>:"Query All Settings.vi"("device type"=w577, "error in (no error)"=w572, "read timeout (500 ms)"=u32 250 ("read timeout (10000 ms)"), "VISA Refnum in"=w569) -> ("error out"=w570:errorcluster, "values"=w579:u32[], "labels"=w578:string[], "checksum ok?"=w573:bool)  [unwired: 3 in, 1 out]
                n296 = case shown="True" w573 {
                  tunnel: w576 -> [_ w594]
                  tunnel: w570 -> [w580 w582]
                  tunnel: [w580 w583] -> w571
                  tunnel: w578 -> [_ w596]
                  tunnel: w579 -> [_ w595]
                  tunnel: w565 -> [_ w581]
                  frame False {
                  }
                  frame True {
                    n297 = local read "settings 4ch"() -> (w584:T4)
                    n298 = local read "delimiter"() -> (w589:string)
                    n299 = call <instrlib>:"Bundle by Name Settings 4ch.vi"("input cluster settings 4ch"=w584, "names"=w596, "values"=w595) -> ("output cluster settings 4ch"=w585:T4)  [unwired: 12 in]
                    n300 = call <vilib>:"Acquire Semaphore.vi"("error in (no error)"=w582, "semaphore"=w581) -> ("error out"=w593:errorcluster, "semaphore out"=w587:T13)  [unwired: 3 in, 1 out]
                    n301 = property on="path-settings" class="Path"(error in=w593) -> (error out=w592:errorcluster, "Value"=w590:path)  [unwired: 1 in, 1 out]
                    n302 = call <instrlib>:"Settings4ch To Settings2ch.vi"("settings4ch"=w585) -> ("settings2ch"=w586:T3)
                    n303 = Get Date/Time In Seconds() -> (seconds since 1Jan1904=w588:timestamp)
                    "timer-settings" <- w588
                    n304 = local write "settings 2ch"(w586) -> ()
                    n305 = local write "settings_old"(w585) -> ()
                    n306 = local write "settings 4ch"(w585) -> ()
                    n307 = call <instrlib>:"writeSettingsFile4ch.vi"("delimiter (,)"=w589, "timestamp (current)"=w588, "error in (no error)"=w592, "old settings"=w594, "new settings"=w585, "path"=w590) -> ("error out"=w591:errorcluster)  [unwired: 4 in, 1 out]
                    n308 = call <vilib>:"Release Semaphore.vi"("error in (no error)"=w591, "semaphore"=w587) -> ("error out"=w583:errorcluster)  [unwired: 4 in, 1 out]
                  }
                }
                n309 = property on="error" class="Clust (strict)"("Val(Sgnl)"=w571) -> (error out=w568:errorcluster)  [unwired: 2 in, 1 out]
                n310 = call <vilib>:"Release Semaphore.vi"("error in (no error)"=w568, "semaphore"=w567) -> ()  [unwired: 4 in, 2 out]
              }
            }
          }
          frame "handle error" {
            n311 = Get Date/Time In Seconds() -> (seconds since 1Jan1904=w610:timestamp)
            n312 = local write "timer-reconnect"(w610) -> ()
            n313 = Flush Queue(queue=w617, error in (no error)=w615) -> (queue out=w616:refnum<queue>, error out=w614:errorcluster)  [unwired: 1 out]
            n314 = local read "error"() -> (w619:errorcluster)
            n315 = Enqueue Element(queue=w616, element="stop acquisition", error in (no error)=w614) -> (queue out=w606:refnum<queue>, error out=w605:errorcluster)  [unwired: 1 in, 1 out]
            n316 = Unbundle By Name(w619) -> ("code"=w618:i32, "source"=w612:string)
            n317 = Enqueue Element(queue=w606, element="disconnect", error in (no error)=w605) -> ()  [unwired: 1 in, 3 out]
            n318 = case shown="Default" w618 {
              tunnel: [w626 w630 w633] -> w604
              tunnel: [errorcluster {"status"=FALSE, "code"=0, "source"=""} ("no error constant") errorcluster {"status"=FALSE, "code"=0, "source"=""} ("no error constant") errorcluster {"status"=FALSE, "code"=0, "source"=""} ("no error constant")] -> w613
              tunnel: w612 -> [_ _ _]
              frame Default {
                w626 = "Connection lost." ("element")
                n319 = property on="status" class="Str"("Text.TextColor"=u32 16744448) -> ()  [unwired: 2 in, 2 out]
                n320 = call <instrlib>:"prependTimestamp.vi"("string in"=w626) -> ("string out"=→"status":string)  [unwired: 14 in]
              }
              frame 0 {
                n321 = disable-structure shown="Enabled" {
                  disable-tunnel: [w631 _] -> w630
                  frame Disabled {
                    w631 = "unknown error" ("message")
                    n322 = One Button Dialog(message=w631) -> ()  [unwired: 1 in, 1 out]
                  }
                  frame Enabled {
                    # "error code 0: unknown error source"
                  }
                }
              }
              frame -1073807360 {
                w633 = "Fatal Error. An error occurred at the communication port. Port is either closed or disconnected."
                n323 = One Button Dialog(message=w633) -> ()  [unwired: 1 in, 1 out]
              }
            }
            n324 = local read "connection state"() -> (w611:T8)
            n325 = case shown="\"connection error\"" w611 {
              selector: w611 -> [w620 _ _ w623 w624]
              tunnel: [w620 connectionState."connection error" ("connection state") connectionState."acquisition error" ("connection state") w623 w624] -> w609
              frame "disconnected", Default {
              }
              frame "connected" {
              }
              frame "acquiring data" {
              }
              frame "connection error" {
              }
              frame "acquisition error" {
              }
            }
            n326 = local write "error"(w613) -> ()
            n327 = call <vilib>:"Acquire Semaphore.vi"("semaphore"=w598) -> ("error out"=w603:errorcluster, "semaphore out"=w602:T13)  [unwired: 4 in, 1 out]
            n328 = local read "delimiter"() -> (w597:string)
            n329 = property on="path-settings" class="Path"(error in=w603) -> (error out=w600:errorcluster, "Value"=w599:path)  [unwired: 1 in, 1 out]
            n330 = local write "connection state"(w609) -> ()
            n331 = call <instrlib>:"writeSettingsFile4ch.vi"("delimiter (,)"=w597, "message (overrides settings)"=w604, "error in (no error)"=w600, "path"=w599) -> ("error out"=w601:errorcluster)  [unwired: 6 in, 1 out]
            n332 = call <vilib>:"Release Semaphore.vi"("error in (no error)"=w601, "semaphore"=w602) -> ()  [unwired: 4 in, 2 out]
          }
          frame "initialize" {
            n333 = disable-structure shown="RUN_TIME_ENGINE==True" {
              frame condition #0 (active) {
                n334 = property on="butExit" class="Bool (strict)"("Visible"=TRUE) -> ()  [unwired: 2 in, 2 out]
              }
              frame condition #1 {
                n335 = property on="butExit" class="Bool (strict)"("Visible"=FALSE) -> ()  [unwired: 2 in, 2 out]
              }
            }
            n336 = Enqueue Element(queue=w651, element="reset controls", error in (no error)=w650) -> (queue out=w635:refnum<queue>, error out=w638:errorcluster)  [unwired: 1 in, 1 out]
            n337 = Enqueue Element(queue=w635, element="reset indicators", error in (no error)=w638) -> (queue out=w636:refnum<queue>, error out=w637:errorcluster)  [unwired: 1 in, 1 out]
            n338 = Enqueue Element(queue=w636, element="reset values", error in (no error)=w637) -> (queue out=w647:refnum<queue>, error out=w648:errorcluster)  [unwired: 1 in, 1 out]
            n339 = Enqueue Element(queue=w647, element="reset timers", error in (no error)=w648) -> (queue out=w641:refnum<queue>, error out=w643:errorcluster)  [unwired: 1 in, 1 out]
            n340 = Enqueue Element(queue=w641, element="create settings file", error in (no error)=w643) -> (queue out=w640:refnum<queue>, error out=w642:errorcluster)  [unwired: 1 in, 1 out]
            n341 = Enqueue Element(queue=w640, element="connect", error in (no error)=w642) -> ()  [unwired: 1 in, 3 out]
          }
          frame "lock settings" {
            n342 = local read "device type"() -> (w655:T6)
            n343 = call <instrlib>:"Get Channels From Device Type.vi"("device type"=w655) -> ("channels"=w654:i32)  [unwired: 4 in]
            n344 = case shown="4, Default" w654 {
              tunnel: T17."Disabled and Grayed Out" ("Disabled") -> [w658 w659]
              frame 4, Default {
                n345 = property on="settings 4ch" class="Clust (strict)"("DisabledEnum"=w658) -> ()  [unwired: 2 in, 2 out]
              }
              frame 2 {
                n346 = property on="settings 2ch" class="Clust (strict)"("DisabledEnum"=w659) -> ()  [unwired: 2 in, 2 out]
              }
            }
            n347 = property on="butUnlockSett" class="Bool"("Visible"=TRUE) -> ()  [unwired: 2 in, 2 out]
          }
          frame "reconnect" {
            n348 = call <vilib>:"Acquire Semaphore.vi"("semaphore"=w664) -> ("error out"=w668:errorcluster, "semaphore out"=w669:T13)  [unwired: 4 in, 1 out]
            n349 = local read "abacus VISA"() -> (w665:refnum<visa-resource-name>)
            n350 = call <instrlib>:"Find Devices.vi"("error in (no error)"=w668) -> ("error out"=w661:errorcluster, "Abacus VISAs"=w667:refnum<visa-resource-name>[])  [unwired: 8 in, 1 out]
            n351 = Search 1D Array(1D array=w667, element=w665) -> (index of element=w666:i32)  [unwired: 1 in]
            n352 = Less Than 0?(x=w666) -> (x < 0?=w663:bool)
            n353 = call <vilib>:"Release Semaphore.vi"("error in (no error)"=w661, "semaphore"=w669) -> ()  [unwired: 4 in, 2 out]
            n354 = case "connection still lost?" shown="False" w663 {
              tunnel: w662 -> [w674 _]
              tunnel: [w671 _] -> w660
              frame False {
                # "when port is back"
                n355 = Flush Queue(queue=w674) -> (queue out=w673:refnum<queue>, error out=w672:errorcluster)  [unwired: 1 in, 1 out]
                n356 = Enqueue Element(queue=w673, element="reconnect step 2", error in (no error)=w672) -> (error out=w671:errorcluster)  [unwired: 1 in, 2 out]
              }
              frame True {
                # "do nothing if port not found"
              }
            }
            n357 = flat-sequence {
              tunnel: w660 -> [_]
              frame #0 {
                n358 = Get Date/Time In Seconds() -> (seconds since 1Jan1904=→"timer-reconnect":timestamp)
              }
            }
          }
          frame "reconnect step 2" {
            n359 = local read "connection state"() -> (w693:T8)
            n360 = local read "abacus VISA"() -> (w678:refnum<visa-resource-name>)
            n361 = call <vilib>:"Acquire Semaphore.vi"("semaphore"=w697) -> ("error out"=w695:errorcluster, "semaphore out"=w694:T13)  [unwired: 4 in, 1 out]
            n362 = call <instrlib>:"Open.vi"("error in (no error)"=w695, "VISA resource name"=w678) -> ("error out"=w696:errorcluster)  [unwired: 8 in, 1 out]
            n363 = call <vilib>:"Release Semaphore.vi"("error in (no error)"=w696, "semaphore"=w694) -> ("error out"=w691:errorcluster)  [unwired: 4 in, 1 out]
            n364 = case shown="\"connection error\"" w693 {
              selector: w693 -> [w698 w699 w700 _ w705]
              tunnel: w692 -> [_ _ _ w703 w714]
              tunnel: w691 -> [_ _ _ w702 w713]
              tunnel: [w698 w699 w700 w701 w705] -> w690
              frame "disconnected", Default {
              }
              frame "connected" {
              }
              frame "acquiring data" {
              }
              frame "connection error" {
                w701 = connectionState."connected" ("connection state")
                n365 = Enqueue Element(queue=w703, element="set settings", error in (no error)=w702) -> ()  [unwired: 1 in, 3 out]
                n366 = local write "connection state"(w701) -> ()
              }
              frame "acquisition error" {
                n367 = Enqueue Element(queue=w714, element="set settings", error in (no error)=w713) -> (queue out=w712:refnum<queue>, error out=w710:errorcluster)  [unwired: 1 in, 1 out]
                n368 = Enqueue Element(queue=w712, element="reset timers", error in (no error)=w710) -> (queue out=w711:refnum<queue>, error out=w709:errorcluster)  [unwired: 1 in, 1 out]
                n369 = Enqueue Element(queue=w711, element="start acquisition", error in (no error)=w709) -> ()  [unwired: 1 in, 3 out]
              }
            }
            n370 = local read "device type"() -> (w676:T6)
            n371 = call <instrlib>:"connectionStatusString.vi"("connected? [T]"=TRUE, "device type"=w676, "Abacus VISA"=w678) -> ("String"=w679:string)  [unwired: 8 in]
            n372 = call <vilib>:"Acquire Semaphore.vi"("semaphore"=w681) -> ("error out"=w686:errorcluster, "semaphore out"=w685:T13)  [unwired: 4 in, 1 out]
            n373 = property on="path-settings" class="Path"(error in=w686) -> (error out=w683:errorcluster, "Value"=w684:path)  [unwired: 1 in, 1 out]
            n374 = local read "delimiter"() -> (w680:string)
            n375 = local read "ref ctrls"() -> (w689:T1)
            n376 = call <instrlib>:"writeSettingsFile4ch.vi"("delimiter (,)"=w680, "message (overrides settings)"=w679, "error in (no error)"=w683, "path"=w684) -> ("error out"=w682:errorcluster)  [unwired: 6 in, 1 out]
            n377 = call <vilib>:"Release Semaphore.vi"("error in (no error)"=w682, "semaphore"=w685) -> ()  [unwired: 4 in, 2 out]
            n378 = call <instrlib>:"prependTimestamp.vi"("string in"=w679) -> ("string out"=w687:string)  [unwired: 14 in]
            n379 = call <instrlib>:"controlVisibility4Ch.vi"("device type [AB1004]"=w676, "ref controls"=w689, "connection state"=w690) -> ()  [unwired: 9 in]
            n380 = property on="status" class="Str"("Text.TextColor"=u32 0, "Value"=w687) -> ()  [unwired: 2 in, 2 out]
          }
          frame "rename files" {
            n381 = call <vilib>:"Acquire Semaphore.vi"("semaphore"=w746) -> ("error out"=w744:errorcluster, "semaphore out"=w745:T13)  [unwired: 4 in, 1 out]
            n382 = property on="path-file" class="Path"(error in=w744) -> (error out=w740:errorcluster, "Value"=w743:path)  [unwired: 1 in, 1 out]
            n383 = property on="path-fileOld" class="Path"(error in=w740, "Value"=w743) -> (error out=w715:errorcluster)  [unwired: 1 in, 1 out]
            n384 = local read "default settings"() -> (w719:T7)
            n385 = property on="path-settings" class="Path"(error in=w715) -> (error out=w717:errorcluster, "Value"=w716:path)  [unwired: 1 in, 1 out]
            n386 = property on="path-settingsOld" class="Path"(error in=w717, "Value"=w716) -> (error out=w731:errorcluster)  [unwired: 1 in, 1 out]
            n387 = Unbundle By Name(w719) -> ("settings_suffix"=w718:string)
            n388 = property on="path-new" class="Path"(error in=w731) -> (error out=w739:errorcluster, "Value"=w742:path)  [unwired: 1 in, 1 out]
            n389 = property on="path-file" class="Path"(error in=w739, "Value"=w742) -> (error out=w738:errorcluster)  [unwired: 1 in, 1 out]
            n390 = call <instrlib>:"settingsSuffixPath.vi"("settings suffix (_settings)"=w718, "path in"=w742) -> ("path out"=w741:path)  [unwired: 2 in]
            n391 = property on="path-settings" class="Path"(error in=w738, "Value"=w741) -> (error out=w727:errorcluster)  [unwired: 1 in, 1 out]
            n392 = property on="path-fileOld" class="Path"(error in=w727) -> ("Value"=w735:path)  [unwired: 1 in, 2 out]
            n393 = property on="path-file" class="Path"(error in=w727) -> (error out=w725:errorcluster, "Value"=w726:path)  [unwired: 1 in, 1 out]
            n394 = call <vilib>:"Is Path and Not Empty.vi"("path"=w735) -> ("Is Path and Not Empty?"=w733:bool)  [unwired: 4 in]
            n395 = call <vilib>:"Check if File or Folder Exists.vi"("error in (no error)"=w725, "path"=w735) -> ("error out"=w730:errorcluster, "file or folder exists?"=w734:bool)  [unwired: 7 in, 1 out]
            n396 = And(x=w733, y=w734) -> (x .and. y?=w737:bool)
            n397 = case "rename file if exists" shown="True" w737 {
              tunnel: w735 -> [_ w756]
              tunnel: w726 -> [_ w755]
              tunnel: w730 -> [w752 w754]
              tunnel: [w752 w753] -> w724
              frame False {
              }
              frame True {
                n398 = Move(source path=w756, error in=w754, 10:w755) -> (error out=w753:errorcluster)  [unwired: 2 in, 2 out]
              }
            }
            n399 = property on="path-settingsOld" class="Path"(error in=w724) -> ("Value"=w732:path)  [unwired: 1 in, 2 out]
            n400 = property on="path-settings" class="Path"(error in=w724) -> (error out=w722:errorcluster, "Value"=w723:path)  [unwired: 1 in, 1 out]
            n401 = call <vilib>:"Check if File or Folder Exists.vi"("error in (no error)"=w722, "path"=w732) -> ("error out"=w729:errorcluster, "file or folder exists?"=w720:bool)  [unwired: 7 in, 1 out]
            n402 = call <vilib>:"Is Path and Not Empty.vi"("path"=w732) -> ("Is Path and Not Empty?"=w721:bool)  [unwired: 4 in]
            n403 = And(x=w721, y=w720) -> (x .and. y?=w736:bool)
            n404 = case "rename file if exists" shown="True" w736 {
              tunnel: w723 -> [_ w751]
              tunnel: w732 -> [_ w750]
              tunnel: w729 -> [w747 w749]
              tunnel: [w747 w748] -> w728
              frame False {
              }
              frame True {
                n405 = Move(source path=w750, error in=w749, 10:w751) -> (error out=w748:errorcluster)  [unwired: 2 in, 2 out]
              }
            }
            n406 = call <vilib>:"Release Semaphore.vi"("error in (no error)"=w728, "semaphore"=w745) -> ()  [unwired: 4 in, 2 out]
          }
          frame "reset controls" {
            w768 = connectionState."disconnected" ("connection state")
            n407 = control-ref of="butConnect"() -> (w763:refnum<vi>)
            n408 = control-ref of="butDisconnect"() -> (w764:refnum<vi>)
            n409 = control-ref of="butStartAcq"() -> (w765:refnum<vi>)
            n410 = control-ref of="butStopAcq"() -> (w766:refnum<vi>)
            n411 = control-ref of="butLoadDefSett"() -> (w762:refnum<vi>)
            n412 = control-ref of="butUnlockSett"() -> (w761:refnum<vi>)
            n413 = control-ref of="settings 2ch"() -> (w758:refnum<vi>)
            n414 = control-ref of="settings 4ch"() -> (w757:refnum<vi>)
            n415 = Bundle(cluster=T1 {"butConnect"=refnum, "butDisconnect"=refnum, "butStartAcq"=refnum, "butStopAcq"=refnum, "butLoadDefSett"=refnum, "butUnlockSett"=refnum, "settings 2ch"=refnum, "settings 4ch"=refnum} ("ref ctrls 2"), "butConnect"=w763, "butDisconnect"=w764, "butStartAcq"=w765, "butStopAcq"=w766, "butLoadDefSett"=w762, "butUnlockSett"=w761, "settings 2ch"=w758, "settings 4ch"=w757) -> (w759:T1)
            "ref ctrls" <- w759
            n416 = local read "device type"() -> (w767:T6)
            n417 = call <instrlib>:"controlVisibility4Ch.vi"("device type [AB1004]"=w767, "ref controls"=w759, "connection state"=w768) -> ()  [unwired: 9 in]
            "connection state" <- w768
          }
          frame "reset indicators" {
            n418 = control-ref of="graph-A"() -> (w775:refnum<vi>)
            n419 = control-ref of="graph-B"() -> (w777:refnum<vi>)
            n420 = control-ref of="graph-C"() -> (w779:refnum<vi>)
            n421 = control-ref of="graph-D"() -> (w781:refnum<vi>)
            n422 = control-ref of="dataTable"() -> (w773:refnum<vi>)
            n423 = control-ref of="counters 2ch"() -> (w769:refnum<vi>)
            n424 = control-ref of="graph coinc"() -> (w774:refnum<vi>)
            n425 = control-ref of="graph-A-S"() -> (w776:refnum<vi>)
            n426 = control-ref of="graph-B-S"() -> (w778:refnum<vi>)
            n427 = control-ref of="graph-C-S"() -> (w780:refnum<vi>)
            n428 = control-ref of="graph-D-S"() -> (w782:refnum<vi>)
            n429 = control-ref of="counters 4ch"() -> (w772:refnum<vi>)
            n430 = Bundle("counters 2ch"=w769, "counters 4ch"=w772, "dataTable"=w773, "graph coinc"=w774, "graph-A"=w775, "graph-A-S"=w776, "graph-B"=w777, "graph-B-S"=w778, "graph-C"=w779, "graph-C-S"=w780, "graph-D"=w781, "graph-D-S"=w782) -> (w771:T2)  [unwired: 1 in]
            "ref indics" <- w771
            n431 = local read "device type"() -> (w770:T6)
            n432 = call <instrlib>:"indicatorVisibility4Ch.vi"("device type [AB1004]"=w770, "ref indics"=w771) -> ()  [unwired: 10 in]
          }
          frame "reset timers" {
            n433 = local read "dataTable"() -> (w784:string[][])
            n434 = local read "settings 4ch"() -> (w791:T4)
            n435 = Empty Array?(array=w784) -> (empty?=w783:bool)
            n436 = Get Date/Time In Seconds() -> (seconds since 1Jan1904=w787:timestamp)
            n437 = case shown="True" w783 {
              tunnel: w787 -> [_ w792]
              frame False {
              }
              frame True {
                "timer-begin" <- w792
              }
            }
            n438 = Unbundle By Name(w791) -> ("sampling"=w789:u32)
            n439 = local write "timer-current"(w787) -> ()
            n440 = local write "timer-lastRead"(w787) -> ()
            n441 = To Double Precision Float(number=w789) -> (double precision float=w788:dbl)
            n442 = Divide(x=w788, y=1000.0) -> (x/y=w786:dbl)
            n443 = Add(x=w787, y=w786) -> (x+y=w785:timestamp)
            n444 = local write "timer-nextRead"(w785) -> ()
          }
          frame "reset values" {
            n445 = stacked-sequence {
              frame #0 {
                w795 = T6 1004 items=["any"=0, "AB1002"=1002, "AB1004"=1004] ("device type")
                # "Clear any data indicators"
                n446 = property on="dataTable" class="Tbl (strict)"("Value"=string[][] [] ("dataTable"), "Index Values"=T19 {"Row"=0, "Column"=0}) -> ()  [unwired: 2 in, 2 out]
                n447 = local write "device type"(w795) -> ()
                n448 = property on="counters 2ch" class="Clust (strict)"("Value"=T10 {"counter_A"=0, "counter_B"=0, "counter_AB"=0, "counters_ID"=0, "time_left"=0} ("counters 2ch")) -> ()  [unwired: 2 in, 2 out]
                n449 = call <instrlib>:"prependTimestamp.vi"("string in"="Session started. Please connect to a device.") -> ("string out"=w798:string)  [unwired: 14 in]
                n450 = local write "error"(errorcluster {"status"=FALSE, "code"=0, "source"=""} ("error constant")) -> ()
                n451 = property on="status" class="Str"("Text.TextColor"=u32 0, "Value"=w798) -> ()  [unwired: 2 in, 2 out]
                n452 = property on="counters 4ch" class="Clust (strict)"("Value"=T18 {"counter_A"=0, "counter_B"=0, "counter_C"=0, "counter_D"=0, "counter_AB"=0, "counter_AC"=0, "counter_AD"=0, "counter_BC"=0, "counter_BD"=0, "counter_CD"=0, "counter_multiple_1"=0, "counters_ID"=0, "time_left"=0}) -> ()  [unwired: 2 in, 2 out]
              }
              frame #1 {
                w803 = cluster{timestamp[], u32[]} {[], []} ("graph-A-S")
                n453 = property on="graph-A-S" class="XYGraph (strict)"("Value"=w803) -> ()  [unwired: 2 in, 2 out]
                n454 = property on="graph-A" class="XYGraph (strict)"("Value"=w803) -> ()  [unwired: 2 in, 2 out]
                n455 = property on="graph-B-S" class="XYGraph (strict)"("Value"=w803) -> ()  [unwired: 2 in, 2 out]
                n456 = property on="graph-B" class="XYGraph (strict)"("Value"=w803) -> ()  [unwired: 2 in, 2 out]
                n457 = property on="graph-C" class="XYGraph (strict)"("Value"=w803) -> ()  [unwired: 2 in, 2 out]
                n458 = property on="graph-C-S" class="XYGraph (strict)"("Value"=w803) -> ()  [unwired: 2 in, 2 out]
                n459 = property on="graph-D" class="XYGraph (strict)"("Value"=w803) -> ()  [unwired: 2 in, 2 out]
                n460 = property on="graph-D-S" class="XYGraph (strict)"("Value"=w803) -> ()  [unwired: 2 in, 2 out]
                n461 = property on="graph coinc" class="XYGraph (strict)"("Value"=cluster{timestamp[], u32[]}[] [] ("graph coinc")) -> ()  [unwired: 2 in, 2 out]
              }
              frame #2 {
                # "'default settings' cluster is set"
                n462 = Current VI's Path() -> (path=w808:path)
                n463 = Strip Path(path=w808) -> (stripped path=w809:path)  [unwired: 1 out]
                n464 = Build Path(base path=w809, name or relative path="settings.py" ("Path")) -> (appended path=w810:path)
                "path-defsettings" <- w810
                n465 = call <vilib>:"Check if File or Folder Exists.vi"("path"=w810) -> ("file or folder exists?"=w806:bool, "dup path"=w807:path)  [unwired: 8 in, 1 out]
                n466 = case shown="True" w806 {
                  tunnel: w807 -> [w812 w814]
                  tunnel: [w811 w813] -> w804
                  frame False {
                    n467 = call <instrlib>:"writeSettingsPy.vi"("Path"=w812) -> ("default settings out"=w811:T7)  [unwired: 9 in, 1 out]
                  }
                  frame True {
                    n468 = call <instrlib>:"readSettingsPy.vi"("Path"=w814) -> ("default settings"=w813:T7)  [unwired: 10 in]
                  }
                }
                n469 = property on="default settings" class="Clust (strict)"("Value"=w804) -> ()  [unwired: 2 in, 2 out]
              }
              frame #3 {
                # "Path construction"
                n470 = local read "default settings"() -> (w817:T7)
                n471 = call <instrlib>:"buildDefaultPath.vi"("default settings"=w817) -> ("settings path"=w815:path, "data path"=w816:path)  [unwired: 3 in]
                n472 = local write "path-file"(w816) -> ()
                n473 = local write "path-settings"(w815) -> ()
              }
              frame #4 {
                n474 = local read "default settings"() -> (w820:T7)
                n475 = Unbundle By Name(w820) -> ("delimiter"=w818:string)
                n476 = case shown="\",\", \";\", Default" w818 {
                  selector: w818 -> [_ _ w823]
                  tunnel: [w821 "\t" w823] -> w819
                  frame "Space", "space" {
                    n477 = call <vilib>:"Space Constant.vi"() -> ("String"=w821:string)
                  }
                  frame "Tab", "tab" {
                  }
                  frame ",", ";", Default {
                  }
                }
                "delimiter" <- w819
              }
              frame #5 {
                n478 = local read "default settings"() -> (w825:T7)
                n479 = Unbundle By Name(w825) -> ("Abacus settings"=w824:T4)
                n480 = call <instrlib>:"Settings4ch To Settings2ch.vi"("settings4ch"=w824) -> ("settings2ch"=w826:T3)
                n481 = local write "settings 2ch"(w826) -> ()
                n482 = local write "settings 4ch"(w824) -> ()
                n483 = local write "settings_old"(w824) -> ()
              }
            }
          }
          frame "set coincidence window" {
            n484 = property on="settings_old" class="Clust (strict)"() -> (error out=w838:errorcluster, "Value"=w827:T4)  [unwired: 2 in, 1 out]
            n485 = call <vilib>:"Acquire Semaphore.vi"("error in (no error)"=w838, "semaphore"=w845) -> ("error out"=w851:errorcluster, "semaphore out"=w852:T13)  [unwired: 3 in, 1 out]
            n486 = local read "abacus VISA"() -> (w850:refnum<visa-resource-name>)
            n487 = local read "device type"() -> (w835:T6)
            n488 = property on="coincidence_window" class="DigNum (strict)"(error in=w851) -> (error out=w849:errorcluster, "Value"=w831:u32)  [unwired: 1 in, 1 out]
            n489 = Format Into String(initial string="Coincidence window set to " ("string in"), w831, "ns." ("string in")) -> (resulting string=w830:string)  [unwired: 2 in, 1 out]
            n490 = call <instrlib>:"Configure Coincidence Window.vi"("device type"=w835, "error in (no error)"=w849, "value ns (10ns)"=w831, "VISA Refnum in"=w850) -> ("error out"=w847:errorcluster, "value ns out"=w848:u32)  [unwired: 5 in, 1 out]
            n491 = call <instrlib>:"prependTimestamp.vi"("string in"=w830) -> ("string out"=w834:string)  [unwired: 14 in]
            n492 = property on="coincidence_window" class="DigNum (strict)"(error in=w847, "Value"=w848) -> (error out=w846:errorcluster)  [unwired: 1 in, 1 out]
            n493 = local write "status"(w834) -> ()
            n494 = call <vilib>:"Release Semaphore.vi"("error in (no error)"=w846, "semaphore"=w852) -> ("error out"=w836:errorcluster)  [unwired: 4 in, 1 out]
            n495 = call <vilib>:"Acquire Semaphore.vi"("semaphore"=w837) -> ("error out"=w844:errorcluster, "semaphore out"=w843:T13)  [unwired: 4 in, 1 out]
            n496 = property on="settings 4ch" class="Clust (strict)"(error in=w836) -> (error out=w829:errorcluster, "Value"=w828:T4)  [unwired: 1 in, 1 out]
            n497 = case shown="No Error" w836 {
              frame No Error {
                n498 = Get Date/Time In Seconds() -> (seconds since 1Jan1904=w853:timestamp)
                n499 = local write "timer-settings"(w853) -> ()
              }
              frame Error {
              }
            }
            n500 = property on="path-settings" class="Path"(error in=w844) -> (error out=w841:errorcluster, "Value"=w840:path)  [unwired: 1 in, 1 out]
            n501 = local read "delimiter"() -> (w839:string)
            n502 = call <instrlib>:"writeSettingsFile4ch.vi"("delimiter (,)"=w839, "error in (no error)"=w841, "old settings"=w827, "new settings"=w828, "path"=w840) -> ("error out"=w842:errorcluster)  [unwired: 5 in, 1 out]
            n503 = property on="settings_old" class="Clust (strict)"(error in=w829, "Value"=w828) -> ()  [unwired: 1 in, 2 out]
            n504 = call <vilib>:"Release Semaphore.vi"("error in (no error)"=w842, "semaphore"=w843) -> ()  [unwired: 4 in, 2 out]
          }
          frame "set default settings" {
            n505 = local read "connection state"() -> (w857:T8)
            n506 = case shown="\"connected\", \"acquiring data\"" w857 {
              tunnel: w856 -> [_ w872]
              tunnel: w855 -> [_ w873]
              tunnel: w854 -> [_ w861]
              frame "disconnected", Default {
              }
              frame "connected", "acquiring data" {
                n507 = local read "default settings"() -> (w878:T7)
                n508 = local read "device type"() -> (w859:T6)
                n509 = property on="settings_old" class="Clust (strict)"(error in=w872) -> (error out=w871:errorcluster, "Value"=w860:T21)  [unwired: 1 in, 1 out]
                n510 = Unbundle By Name(w878) -> ("Abacus settings"=w879:T4)
                n511 = call <instrlib>:"Get Channels From Device Type.vi"("device type"=w859) -> ("channels"=w858:i32)  [unwired: 4 in]
                n512 = case shown="2" w858 {
                  tunnel: w879 -> [w887 w891]
                  tunnel: [w886 w889] -> w880
                  tunnel: [w885 w888] -> w881
                  frame 4, Default {
                    n513 = call <instrlib>:"Unbundle by Name Settings 4ch.vi"("input cluster settings 4ch"=w887) -> ("names"=w885:string[], "values"=w886:u32[])  [unwired: 13 in]
                  }
                  frame 2 {
                    n514 = call <instrlib>:"Settings4ch To Settings2ch.vi"("settings4ch"=w891) -> ("settings2ch"=w890:T3)
                    n515 = call <instrlib>:"Unbundle by Name Settings 2ch.vi"("input cluster settings 2ch"=w890) -> ("names"=w888:string[], "values"=w889:u32[])  [unwired: 13 in]
                  }
                }
                n516 = local read "abacus VISA"() -> (w874:refnum<visa-resource-name>)
                n517 = call <instrlib>:"prependTimestamp.vi"("string in"="Default settings loaded.") -> ("string out"=w882:string)  [unwired: 14 in]
                n518 = local write "status"(w882) -> ()
                n519 = call <vilib>:"Acquire Semaphore.vi"("error in (no error)"=w871, "semaphore"=w873) -> ("error out"=w877:errorcluster, "semaphore out"=w876:T13)  [unwired: 3 in, 1 out]
                n520 = call <instrlib>:"Configure By Name.vi"("device type"=w859, "error in (no error)"=w877, "values"=w880, "labels"=w881, "VISA Refnum in"=w874) -> ("error out"=w875:errorcluster)  [unwired: 5 in, 1 out]
                n521 = local read "delimiter"() -> (w865:string)
                n522 = call <vilib>:"Release Semaphore.vi"("error in (no error)"=w875, "semaphore"=w876) -> ("error out"=w862:errorcluster)  [unwired: 4 in, 1 out]
                n523 = call <vilib>:"Acquire Semaphore.vi"("error in (no error)"=w862, "semaphore"=w861) -> ("error out"=w870:errorcluster, "semaphore out"=w869:T13)  [unwired: 3 in, 1 out]
                n524 = case shown="No Error" w862 {
                  frame No Error {
                    n525 = Get Date/Time In Seconds() -> (seconds since 1Jan1904=w884:timestamp)
                    n526 = local write "timer-settings"(w884) -> ()
                  }
                  frame Error {
                  }
                }
                n527 = property on="path-settings" class="Path"(error in=w870) -> (error out=w867:errorcluster, "Value"=w866:path)  [unwired: 1 in, 1 out]
                n528 = property on="settings 4ch" class="Clust (strict)"(error in=w862) -> (error out=w864:errorcluster, "Value"=w863:T21)  [unwired: 1 in, 1 out]
                n529 = call <instrlib>:"writeSettingsFile4ch.vi"("delimiter (,)"=w865, "error in (no error)"=w867, "old settings"=w860, "new settings"=w863, "path"=w866) -> ("error out"=w868:errorcluster)  [unwired: 5 in, 1 out]
                n530 = property on="settings_old" class="Clust (strict)"(error in=w864, "Value"=w863) -> ()  [unwired: 1 in, 2 out]
                n531 = call <vilib>:"Release Semaphore.vi"("error in (no error)"=w868, "semaphore"=w869) -> ()  [unwired: 4 in, 2 out]
              }
            }
          }
          frame "set delay A".."set delay Z" {
            w914 = T23 0 items=["none", "A", "B", "C", "D", "E", "F", "G", "H"] ("channel")
            n532 = property on="settings_old" class="Clust (strict)"() -> (error out=w902:errorcluster, "Value"=w909:T21)  [unwired: 2 in, 1 out]
            n533 = call <instrlib>:"getLastChar.vi"("string"=w911) -> ("last char"=w892:string)
            n534 = call <instrlib>:"letterToNumber.vi"("letter"=w892) -> ("number"=w913:u8)
            n535 = call <vilib>:"Acquire Semaphore.vi"("error in (no error)"=w902, "semaphore"=w910) -> ("error out"=w920:errorcluster, "semaphore out"=w921:T13)  [unwired: 3 in, 1 out]
            n536 = Type Cast(type=w914, x=w913) -> (*(type *) &x=w912:T23)
            n537 = local read "abacus VISA"() -> (w919:refnum<visa-resource-name>)
            n538 = local read "device type"() -> (w922:T6)
            n539 = case shown="1" w912 {
              tunnel: w920 -> [w937 w940 w943 w946 w949]
              tunnel: [_ w939 w942 w945 w948] -> w918
              tunnel: [w937 w938 w941 w944 w947] -> w917
              frame 0, Default {
              }
              frame 1 {
                n540 = property on="delay_A" class="DigNum (strict)"(error in=w940) -> (error out=w938:errorcluster, "Value"=w939:u32)  [unwired: 1 in, 1 out]
              }
              frame 2 {
                n541 = property on="delay_B" class="DigNum (strict)"(error in=w943) -> (error out=w941:errorcluster, "Value"=w942:u32)  [unwired: 1 in, 1 out]
              }
              frame 3 {
                n542 = property on="delay_C" class="DigNum (strict)"(error in=w946) -> (error out=w944:errorcluster, "Value"=w945:u32)  [unwired: 1 in, 1 out]
              }
              frame 4 {
                n543 = property on="delay_D" class="DigNum (strict)"(error in=w949) -> (error out=w947:errorcluster, "Value"=w948:u32)  [unwired: 1 in, 1 out]
              }
            }
            n544 = call <instrlib>:"Configure Delay.vi"("device type"=w922, "error in (no error)"=w917, "value (0 ns)"=w918, "channel"=w912, "VISA Refnum in"=w919) -> ("error out"=w916:errorcluster, "value ns out"=w894:u32)  [unwired: 4 in, 1 out]
            n545 = Format Into String(initial string="Delay set to " ("string in"), w894, "ns in channel" ("string in"), w892) -> (resulting string=w897:string)  [unwired: 2 in, 1 out]
            n546 = call <instrlib>:"prependTimestamp.vi"("string in"=w897) -> ("string out"=w896:string)  [unwired: 14 in]
            n547 = case shown="1" w912 {
              tunnel: w894 -> [_ w927 w930 w933 w936]
              tunnel: w916 -> [w924 w926 w929 w932 w935]
              tunnel: [w924 w925 w928 w931 w934] -> w915
              frame 0, Default {
              }
              frame 1 {
                n548 = property on="delay_A" class="DigNum (strict)"(error in=w926, "Value"=w927) -> (error out=w925:errorcluster)  [unwired: 1 in, 1 out]
              }
              frame 2 {
                n549 = property on="delay_B" class="DigNum (strict)"(error in=w929, "Value"=w930) -> (error out=w928:errorcluster)  [unwired: 1 in, 1 out]
              }
              frame 3 {
                n550 = property on="delay_C" class="DigNum (strict)"(error in=w932, "Value"=w933) -> (error out=w931:errorcluster)  [unwired: 1 in, 1 out]
              }
              frame 4 {
                n551 = property on="delay_D" class="DigNum (strict)"(error in=w935, "Value"=w936) -> (error out=w934:errorcluster)  [unwired: 1 in, 1 out]
              }
            }
            n552 = local write "status"(w896) -> ()
            n553 = call <vilib>:"Acquire Semaphore.vi"("semaphore"=w901) -> ("error out"=w908:errorcluster, "semaphore out"=w907:T13)  [unwired: 4 in, 1 out]
            n554 = call <vilib>:"Release Semaphore.vi"("error in (no error)"=w915, "semaphore"=w921) -> ("error out"=w898:errorcluster)  [unwired: 4 in, 1 out]
            n555 = case shown="No Error" w898 {
              frame No Error {
                n556 = Get Date/Time In Seconds() -> (seconds since 1Jan1904=w923:timestamp)
                n557 = local write "timer-settings"(w923) -> ()
              }
              frame Error {
              }
            }
            n558 = property on="path-settings" class="Path"(error in=w908) -> (error out=w905:errorcluster, "Value"=w904:path)  [unwired: 1 in, 1 out]
            n559 = local read "delimiter"() -> (w903:string)
            n560 = property on="settings 4ch" class="Clust (strict)"(error in=w898) -> (error out=w900:errorcluster, "Value"=w899:T21)  [unwired: 1 in, 1 out]
            n561 = call <instrlib>:"writeSettingsFile4ch.vi"("delimiter (,)"=w903, "error in (no error)"=w905, "old settings"=w909, "new settings"=w899, "path"=w904) -> ("error out"=w906:errorcluster)  [unwired: 5 in, 1 out]
            n562 = property on="settings_old" class="Clust (strict)"(error in=w900, "Value"=w899) -> ()  [unwired: 1 in, 2 out]
            n563 = call <vilib>:"Release Semaphore.vi"("error in (no error)"=w906, "semaphore"=w907) -> ()  [unwired: 4 in, 2 out]
          }
          frame "set multi 1".."set multi 9" {
            w969 = u8 0  # U8
            n564 = property on="settings_old" class="Clust (strict)"() -> (error out=w958:errorcluster, "Value"=w965:T21)  [unwired: 2 in, 1 out]
            n565 = property on="config_multiple_1" class="Ring (strict)"() -> ("RingText.Text"=w952:string)  [unwired: 2 in, 2 out]
            n566 = call <instrlib>:"getLastChar.vi"("string"=w966) -> ("last char"=w970:string)
            n567 = Decimal String To Number(string=w970, default (0L)=w969) -> (number=w975:u8)  [unwired: 1 in, 1 out]
            n568 = call <vilib>:"Acquire Semaphore.vi"("error in (no error)"=w958, "semaphore"=w967) -> ("error out"=w972:errorcluster, "semaphore out"=w971:T13)  [unwired: 3 in, 1 out]
            n569 = case shown="1" w975 {
              tunnel: w972 -> [w984 w987]
              tunnel: [w984 w986] -> w973
              tunnel: [_ w985] -> w974
              frame 0, Default {
              }
              frame 1 {
                n570 = property on="config_multiple_1" class="Ring (strict)"(error in=w987) -> (error out=w986:errorcluster, "Value"=w985:T22)  [unwired: 1 in, 1 out]
              }
            }
            n571 = Concatenate Strings("Multi-fold set to " ("string in"), w952) -> (w953:string)
            n572 = case shown="1..8" w975 {
              selector: w975 -> [_ w978]
              tunnel: [w977 w983] -> w968
              tunnel: w973 -> [w977 w980]
              tunnel: w974 -> [_ w979]
              frame 0, Default {
              }
              frame 1..8 {
                n573 = local read "abacus VISA"() -> (w981:refnum<visa-resource-name>)
                n574 = local read "device type"() -> (w982:T6)
                n575 = call <instrlib>:"Configure Multiple Coincidence.vi"("device type"=w982, "error in (no error)"=w980, "Multiple coincidence configuration"=w979, "multi-fold counter (1)"=w978, "VISA Refnum in"=w981) -> ("error out"=w983:errorcluster)  [unwired: 5 in, 1 out]
              }
            }
            n576 = call <instrlib>:"prependTimestamp.vi"("string in"=w953) -> ("string out"=w950:string)  [unwired: 14 in]
            n577 = local write "status"(w950) -> ()
            n578 = call <vilib>:"Acquire Semaphore.vi"("semaphore"=w957) -> ("error out"=w964:errorcluster, "semaphore out"=w963:T13)  [unwired: 4 in, 1 out]
            n579 = call <vilib>:"Release Semaphore.vi"("error in (no error)"=w968, "semaphore"=w971) -> ("error out"=w955:errorcluster)  [unwired: 4 in, 1 out]
            n580 = case shown="No Error" w955 {
              frame No Error {
                n581 = Get Date/Time In Seconds() -> (seconds since 1Jan1904=w976:timestamp)
                n582 = local write "timer-settings"(w976) -> ()
              }
              frame Error {
              }
            }
            n583 = property on="path-settings" class="Path"(error in=w964) -> (error out=w961:errorcluster, "Value"=w960:path)  [unwired: 1 in, 1 out]
            n584 = local read "delimiter"() -> (w959:string)
            n585 = property on="settings 4ch" class="Clust (strict)"(error in=w955) -> (error out=w956:errorcluster, "Value"=w954:T21)  [unwired: 1 in, 1 out]
            n586 = call <instrlib>:"writeSettingsFile4ch.vi"("delimiter (,)"=w959, "error in (no error)"=w961, "old settings"=w965, "new settings"=w954, "path"=w960) -> ("error out"=w962:errorcluster)  [unwired: 5 in, 1 out]
            n587 = property on="settings_old" class="Clust (strict)"(error in=w956, "Value"=w954) -> ()  [unwired: 1 in, 2 out]
            n588 = call <vilib>:"Release Semaphore.vi"("error in (no error)"=w962, "semaphore"=w963) -> ()  [unwired: 4 in, 2 out]
          }
          frame "set sampling" {
            n589 = property on="settings_old" class="Clust (strict)"() -> (error out=w1000:errorcluster, "Value"=w997:T21)  [unwired: 2 in, 1 out]
            n590 = call <vilib>:"Acquire Semaphore.vi"("error in (no error)"=w1000, "semaphore"=w1007) -> ("error out"=w1012:errorcluster, "semaphore out"=w1013:T13)  [unwired: 3 in, 1 out]
            n591 = local read "abacus VISA"() -> (w1011:refnum<visa-resource-name>)
            n592 = local read "device type"() -> (w994:T6)
            n593 = property on="sampling" class="Ring (strict)"(error in=w1012) -> (error out=w1009:errorcluster, "Value"=w1010:u32)  [unwired: 1 in, 1 out]
            n594 = call <instrlib>:"Configure Sampling Time.vi"("device type"=w994, "error in (no error)"=w1009, "value (1000 ms)"=w1010, "VISA Refnum in"=w1011) -> ("error out"=w1008:errorcluster, "value ms out"=w989:u32)  [unwired: 5 in, 1 out]
            n595 = Format Into String(initial string="Sampling set to " ("string in"), w989, "ms." ("string in")) -> (resulting string=w993:string)  [unwired: 2 in, 1 out]
            n596 = call <instrlib>:"prependTimestamp.vi"("string in"=w993) -> ("string out"=w992:string)  [unwired: 14 in]
            n597 = property on="sampling" class="Ring (strict)"(error in=w1008, "Value"=w989) -> (error out=w998:errorcluster)  [unwired: 1 in, 1 out]
            n598 = local write "status"(w992) -> ()
            n599 = call <vilib>:"Release Semaphore.vi"("error in (no error)"=w998, "semaphore"=w1013) -> ("error out"=w996:errorcluster)  [unwired: 4 in, 1 out]
            n600 = call <vilib>:"Acquire Semaphore.vi"("semaphore"=w999) -> ("error out"=w1006:errorcluster, "semaphore out"=w1005:T13)  [unwired: 4 in, 1 out]
            n601 = property on="settings 4ch" class="Clust (strict)"(error in=w996) -> (error out=w995:errorcluster, "Value"=w988:T21)  [unwired: 1 in, 1 out]
            n602 = property on="path-settings" class="Path"(error in=w1006) -> (error out=w1003:errorcluster, "Value"=w1002:path)  [unwired: 1 in, 1 out]
            n603 = local read "delimiter"() -> (w1001:string)
            n604 = case shown="No Error" w996 {
              frame No Error {
                n605 = Get Date/Time In Seconds() -> (seconds since 1Jan1904=w1014:timestamp)
                n606 = local write "timer-settings"(w1014) -> ()
              }
              frame Error {
              }
            }
            n607 = call <instrlib>:"writeSettingsFile4ch.vi"("delimiter (,)"=w1001, "error in (no error)"=w1003, "old settings"=w997, "new settings"=w988, "path"=w1002) -> ("error out"=w1004:errorcluster)  [unwired: 5 in, 1 out]
            n608 = property on="settings_old" class="Clust (strict)"(error in=w995, "Value"=w988) -> ()  [unwired: 1 in, 2 out]
            n609 = call <vilib>:"Release Semaphore.vi"("error in (no error)"=w1004, "semaphore"=w1005) -> ()  [unwired: 4 in, 2 out]
          }
          frame "set settings" {
            n610 = local read "device type"() -> (w1016:T6)
            n611 = call <instrlib>:"Get Channels From Device Type.vi"("device type"=w1016) -> ("channels"=w1015:i32)  [unwired: 4 in]
            n612 = case shown="4, Default" w1015 {
              tunnel: [string[] ["set sampling", "set coincidence window", "set delay A", "set delay B", "set delay C", "set delay D", "set sleep A", "set sleep B", "set sleep C", "set sleep D", "set multi 1"] string[] ["set sampling", "set coincidence window", "set delay A", "set delay B", "set sleep A", "set sleep B"]] -> w1019
              frame 4, Default {
              }
              frame 2 {
              }
            }
            n613 = for {
              tunnel: w1019 -> [w1022] mode=indexing
              shift-right: [w1025] -> _
              shift-left: w1017 -> [w1026]
              shift-right: [w1023] -> _
              shift-left: w1018 -> [w1024]
              n614 = Enqueue Element(queue=w1024, element=w1022, error in (no error)=w1026) -> (queue out=w1023:refnum<queue>, error out=w1025:errorcluster)  [unwired: 1 in, 1 out]
            }
          }
          frame "set sleep A".."set sleep Z" {
            w1049 = T23 0 items=["none", "A", "B", "C", "D", "E", "F", "G", "H"] ("channel")
            n615 = call <instrlib>:"getLastChar.vi"("string"=w1046) -> ("last char"=w1027:string)
            n616 = property on="settings_old" class="Clust (strict)"() -> (error out=w1037:errorcluster, "Value"=w1044:T21)  [unwired: 2 in, 1 out]
            n617 = call <instrlib>:"letterToNumber.vi"("letter"=w1027) -> ("number"=w1048:u8)
            n618 = Type Cast(type=w1049, x=w1048) -> (*(type *) &x=w1047:T23)
            n619 = call <vilib>:"Acquire Semaphore.vi"("error in (no error)"=w1037, "semaphore"=w1045) -> ("error out"=w1055:errorcluster, "semaphore out"=w1056:T13)  [unwired: 3 in, 1 out]
            n620 = local read "abacus VISA"() -> (w1054:refnum<visa-resource-name>)
            n621 = local read "device type"() -> (w1057:T6)
            n622 = case shown="1" w1047 {
              tunnel: w1055 -> [w1072 w1075 w1078 w1081 w1084]
              tunnel: [_ w1074 w1077 w1080 w1083] -> w1053
              tunnel: [w1072 w1073 w1076 w1079 w1082] -> w1052
              frame 0, Default {
              }
              frame 1 {
                n623 = property on="sleep_A" class="DigNum (strict)"(error in=w1075) -> (error out=w1073:errorcluster, "Value"=w1074:u32)  [unwired: 1 in, 1 out]
              }
              frame 2 {
                n624 = property on="sleep_B" class="DigNum (strict)"(error in=w1078) -> (error out=w1076:errorcluster, "Value"=w1077:u32)  [unwired: 1 in, 1 out]
              }
              frame 3 {
                n625 = property on="sleep_C" class="DigNum (strict)"(error in=w1081) -> (error out=w1079:errorcluster, "Value"=w1080:u32)  [unwired: 1 in, 1 out]
              }
              frame 4 {
                n626 = property on="sleep_D" class="DigNum (strict)"(error in=w1084) -> (error out=w1082:errorcluster, "Value"=w1083:u32)  [unwired: 1 in, 1 out]
              }
            }
            n627 = call <instrlib>:"Configure Sleep.vi"("device type"=w1057, "error in (no error)"=w1052, "value (0 ns)"=w1053, "channel"=w1047, "VISA Refnum in"=w1054) -> ("error out"=w1051:errorcluster, "value ns out"=w1028:u32)  [unwired: 4 in, 1 out]
            n628 = Format Into String(initial string="Sleep time set to " ("string in"), w1028, "ns in channel" ("string in"), w1027) -> (resulting string=w1032:string)  [unwired: 2 in, 1 out]
            n629 = call <instrlib>:"prependTimestamp.vi"("string in"=w1032) -> ("string out"=w1031:string)  [unwired: 14 in]
            n630 = local write "status"(w1031) -> ()
            n631 = case shown="1" w1047 {
              tunnel: w1028 -> [_ w1062 w1065 w1068 w1071]
              tunnel: w1051 -> [w1059 w1061 w1064 w1067 w1070]
              tunnel: [w1059 w1060 w1063 w1066 w1069] -> w1050
              frame 0, Default {
              }
              frame 1 {
                n632 = property on="sleep_A" class="DigNum (strict)"(error in=w1061, "Value"=w1062) -> (error out=w1060:errorcluster)  [unwired: 1 in, 1 out]
              }
              frame 2 {
                n633 = property on="sleep_B" class="DigNum (strict)"(error in=w1064, "Value"=w1065) -> (error out=w1063:errorcluster)  [unwired: 1 in, 1 out]
              }
              frame 3 {
                n634 = property on="sleep_C" class="DigNum (strict)"(error in=w1067, "Value"=w1068) -> (error out=w1066:errorcluster)  [unwired: 1 in, 1 out]
              }
              frame 4 {
                n635 = property on="sleep_D" class="DigNum (strict)"(error in=w1070, "Value"=w1071) -> (error out=w1069:errorcluster)  [unwired: 1 in, 1 out]
              }
            }
            n636 = call <vilib>:"Acquire Semaphore.vi"("semaphore"=w1036) -> ("error out"=w1043:errorcluster, "semaphore out"=w1042:T13)  [unwired: 4 in, 1 out]
            n637 = call <vilib>:"Release Semaphore.vi"("error in (no error)"=w1050, "semaphore"=w1056) -> ("error out"=w1035:errorcluster)  [unwired: 4 in, 1 out]
            n638 = case shown="No Error" w1035 {
              frame No Error {
                n639 = Get Date/Time In Seconds() -> (seconds since 1Jan1904=w1058:timestamp)
                n640 = local write "timer-settings"(w1058) -> ()
              }
              frame Error {
              }
            }
            n641 = property on="path-settings" class="Path"(error in=w1043) -> (error out=w1040:errorcluster, "Value"=w1039:path)  [unwired: 1 in, 1 out]
            n642 = local read "delimiter"() -> (w1038:string)
            n643 = property on="settings 4ch" class="Clust (strict)"(error in=w1035) -> (error out=w1033:errorcluster, "Value"=w1034:T21)  [unwired: 1 in, 1 out]
            n644 = call <instrlib>:"writeSettingsFile4ch.vi"("delimiter (,)"=w1038, "error in (no error)"=w1040, "old settings"=w1044, "new settings"=w1034, "path"=w1039) -> ("error out"=w1041:errorcluster)  [unwired: 5 in, 1 out]
            n645 = property on="settings_old" class="Clust (strict)"(error in=w1033, "Value"=w1034) -> ()  [unwired: 1 in, 2 out]
            n646 = call <vilib>:"Release Semaphore.vi"("error in (no error)"=w1041, "semaphore"=w1042) -> ()  [unwired: 4 in, 2 out]
          }
          frame "start acquisition" {
            w1097 = connectionState."acquiring data" ("connection state")
            n647 = local read "device type"() -> (w1085:T6)
            n648 = local read "dataTable"() -> (w1099:string[][])
            n649 = Empty Array?(array=w1099) -> (empty?=w1098:bool)
            n650 = local read "ref ctrls"() -> (w1096:T1)
            n651 = local write "connection state"(w1097) -> ()
            n652 = case shown="True" w1098 {
              tunnel: ["Acquisition started." "Acquisition started. Current time is 0s."] -> w1094
              tunnel: [w1100 w1103] -> w1093
              frame False {
                n653 = Get Date/Time In Seconds() -> (seconds since 1Jan1904=w1100:timestamp)
              }
              frame True {
                n654 = local read "timer-begin"() -> (w1103:timestamp)
              }
            }
            n655 = call <instrlib>:"controlVisibility4Ch.vi"("device type [AB1004]"=w1085, "ref controls"=w1096, "connection state"=w1097) -> ()  [unwired: 9 in]
            n656 = call <vilib>:"Acquire Semaphore.vi"("semaphore"=w1087) -> ("error out"=w1092:errorcluster, "semaphore out"=w1091:T13)  [unwired: 4 in, 1 out]
            n657 = property on="path-settings" class="Path"(error in=w1092) -> (error out=w1089:errorcluster, "Value"=w1088:path)  [unwired: 1 in, 1 out]
            n658 = local read "delimiter"() -> (w1086:string)
            n659 = call <instrlib>:"prependTimestamp.vi"("string in"=w1094) -> ("string out"=w1095:string)  [unwired: 14 in]
            n660 = call <instrlib>:"writeSettingsFile4ch.vi"("delimiter (,)"=w1086, "message (overrides settings)"=w1094, "timestamp (current)"=w1093, "error in (no error)"=w1089, "path"=w1088) -> ("error out"=w1090:errorcluster)  [unwired: 5 in, 1 out]
            n661 = local write "status"(w1095) -> ()
            n662 = call <vilib>:"Release Semaphore.vi"("error in (no error)"=w1090, "semaphore"=w1091) -> ()  [unwired: 4 in, 2 out]
          }
          frame "stop acquisition" {
            w1112 = "Acquisition stopped."
            n663 = local read "connection state"() -> (w1115:T8)
            n664 = case shown="\"acquiring data\", Default" w1115 {
              selector: w1115 -> [_ w1119 w1120]
              tunnel: [connectionState."connected" ("connection state") w1119 w1120] -> w1114
              tunnel: w1112 -> [w1116 _ _]
              frame "acquiring data", Default {
                n665 = call <instrlib>:"prependTimestamp.vi"("string in"=w1116) -> ("string out"=w1117:string)  [unwired: 14 in]
                n666 = local write "status"(w1117) -> ()
              }
              frame "connection error" {
              }
              frame "acquisition error" {
              }
            }
            n667 = call <vilib>:"Acquire Semaphore.vi"("semaphore"=w1106) -> ("error out"=w1111:errorcluster, "semaphore out"=w1110:T13)  [unwired: 4 in, 1 out]
            n668 = local read "delimiter"() -> (w1105:string)
            n669 = property on="path-settings" class="Path"(error in=w1111) -> (error out=w1108:errorcluster, "Value"=w1107:path)  [unwired: 1 in, 1 out]
            n670 = call <instrlib>:"writeSettingsFile4ch.vi"("delimiter (,)"=w1105, "message (overrides settings)"=w1112, "error in (no error)"=w1108, "path"=w1107) -> ("error out"=w1109:errorcluster)  [unwired: 6 in, 1 out]
            n671 = local write "connection state"(w1114) -> ()
            n672 = local read "ref ctrls"() -> (w1113:T1)
            n673 = call <vilib>:"Release Semaphore.vi"("error in (no error)"=w1109, "semaphore"=w1110) -> ()  [unwired: 4 in, 2 out]
            n674 = local read "device type"() -> (w1104:T6)
            n675 = call <instrlib>:"controlVisibility4Ch.vi"("device type [AB1004]"=w1104, "ref controls"=w1113, "connection state"=w1114) -> ()  [unwired: 9 in]
          }
          frame "unlock settings" {
            n676 = local read "device type"() -> (w1122:T6)
            n677 = call <instrlib>:"Get Channels From Device Type.vi"("device type"=w1122) -> ("channels"=w1121:i32)  [unwired: 4 in]
            n678 = property on="butUnlockSett" class="Bool"("Visible"=FALSE) -> (error out=w1123:errorcluster)  [unwired: 2 in, 1 out]
            n679 = case shown="4, Default" w1121 {
              tunnel: T17."Enabled" ("Disabled") -> [w1127 w1128]
              frame 4, Default {
                n680 = property on="settings 4ch" class="Clust (strict)"("DisabledEnum"=w1127) -> ()  [unwired: 2 in, 2 out]
              }
              frame 2 {
                n681 = property on="settings 2ch" class="Clust (strict)"("DisabledEnum"=w1128) -> ()  [unwired: 2 in, 2 out]
              }
            }
            n682 = property on="butLoadDefSett" class="Bool"(error in=w1123, "Visible"=TRUE) -> ()  [unwired: 1 in, 2 out]
          }
          frame Default {
          }
        }
      }
      frame Error {
        # "Return true in any case that should stop the loop."
      }
    }
  }
  n683 = while {
    tunnel: w15 -> [w1138]
    tunnel: w17 -> [w1134]
    tunnel: w16 -> [w1133]
    stop <- w1137 stop-if-true
    # "read sample loop"
    n684 = Wait on Notification(notifier=w1138, ignore previous (F)=TRUE) -> (notification=w1136:timestamp, error out=w1130:errorcluster)  [unwired: 2 in, 2 out]
    n685 = local read "error"() -> (w1132:errorcluster)
    n686 = Merge Errors(w1130, w1132) -> (w1131:errorcluster)
    n687 = case shown="No Error" w1131 {
      tunnel: [FALSE w1163] -> w1137
      tunnel: w1136 -> [w1155 _]
      tunnel: w1134 -> [w1157 _]
      tunnel: w1133 -> [w1156 _]
      tunnel: w1130 -> [_ w1164]
      frame No Error {
        n688 = local read "abacus VISA"() -> (w1150:refnum<visa-resource-name>)
        n689 = local read "device type"() -> (w1139:T6)
        n690 = call <vilib>:"Acquire Semaphore.vi"("semaphore"=w1156) -> ("error out"=w1152:errorcluster, "semaphore out"=w1154:T13)  [unwired: 4 in, 1 out]
        n691 = call <instrlib>:"Read Measurement.vi"("device type"=w1139, "error in (no error)"=w1152, "read timeout (500 ms)"=u32 250 ("read timeout (10000 ms)"), "VISA Refnum in"=w1150) -> ("error out"=w1151:errorcluster, "values"=w1141:u32[], "labels"=w1142:string[], "read time"=w1148:timestamp)  [unwired: 2 in, 2 out]
        "timer-lastRead" <- w1148
        n692 = property on="error" class="Clust (strict)"("Val(Sgnl)"=w1151) -> (error out=w1153:errorcluster)  [unwired: 2 in, 1 out]
        n693 = call <instrlib>:"Bundle by Name Data 4ch.vi"("names"=w1142, "values"=w1141) -> ("output cluster 4ch"=w1140:T11)  [unwired: 13 in]
        n694 = call <vilib>:"Release Semaphore.vi"("error in (no error)"=w1153, "semaphore"=w1154) -> ()  [unwired: 4 in, 2 out]
        n695 = Unbundle By Name(w1140) -> ("counters_ID"=w1143:u32)
        n696 = Unbundle By Name(w1140) -> ("time_left"=w1145:u32)
        n697 = Divide(x=w1145, y=1000.0) -> (x/y=w1144:dbl)
        n698 = case shown="1.." w1143 {
          tunnel: w1157 -> [w1162 _]
          tunnel: w1140 -> [w1161 _]
          tunnel: w1148 -> [w1160 _]
          frame 1.. {
            n699 = Bundle("read time"=w1160, "output cluster 4ch"=w1161) -> (w1159:T24)  [unwired: 1 in]
            n700 = Enqueue Element "adds data in queue"(queue=w1162, element=w1159) -> ()  [unwired: 2 in, 3 out]
          }
          frame 0, Default {
            # "ID=0 means\ninvalid data"
          }
        }
        n701 = Add(x=w1148, y=w1144) -> (x+y=→"timer-nextRead":timestamp)
        "timer-readRequest" <- w1155
      }
      frame Error {
        n702 = Unbundle By Name(w1164) -> ("status"=w1163:bool)
      }
    }
  }
  n703 = while {
    tunnel: w14 -> [w1171]
    tunnel: w12 -> [w1169]
    shift-right: [w1168] -> _
    shift-left: w2 -> [w1167]
    shift-right: [w1165] -> _
    shift-left: w1 -> [w1166]
    stop <- w1173 stop-if-true
    w1172 = u32 250  # refresh rate
    # "update dataGUI and datafile loop"
    n704 = Dequeue Element(queue=w1171) -> (queue out=w1170:refnum<queue>, element=w1175:T15, error out=w1174:errorcluster)  [unwired: 2 in, 1 out]
    n705 = Wait (ms)(milliseconds to wait=w1172) -> ()  [unwired: 1 out]
    n706 = case shown="No Error" w1174 {
      selector: w1174 -> [w1215 _]
      tunnel: w1175 -> [w1214 _]
      tunnel: [FALSE TRUE] -> w1173
      tunnel: w1170 -> [w1216 _]
      tunnel: w1169 -> [w1208 _]
      tunnel: [w1185 w1219] -> w1168
      tunnel: w1167 -> [w1194 w1219]
      tunnel: w1166 -> [w1180 w1218]
      tunnel: [w1179 w1218] -> w1165
      frame No Error {
        w1186 = 100  # data in graphs
        n707 = Flush Queue(queue=w1216, error in (no error)=w1215) -> (remaining elements=w1213:T12)  [unwired: 2 out]
        n708 = local read "timer-begin"() -> (w1197:timestamp)
        n709 = local read "device type"() -> (w1176:T6)
        n710 = Build Array (concatenate)(w1214, w1213) -> (w1210:T12)
        n711 = Reverse 1D Array "most\nrecent first"(array=w1210) -> (reversed array=w1195:T12)
        n712 = call <instrlib>:"timestampAndDataToTable 4ch.vi"("device type [AB1004]"=w1176, "data in"=w1195, "session start timestamp"=w1197) -> ("table data"=w1178:string[][], "table headers"=w1196:string[])  [unwired: 6 in, 1 out]
        n713 = local read "delimiter"() -> (w1200:string)
        n714 = Index Array "get most\nrecent value"(array=w1195, index=0) -> (element=w1211:T15)
        n715 = property on="dataTable" class="Tbl (strict)"("Column Headers[]"=w1196) -> ()  [unwired: 2 in, 2 out]
        n716 = Build Array (concatenate) "prepend new data"(w1195, w1194) -> (w1187:T12)
        n717 = Build Array (concatenate) "prepend new data"(w1178, w1180) -> (w1179:string[][])
        "dataTable" <- w1179
        n718 = call <vilib>:"reverse 2D array.vi"("Previously Selected List"=w1178) -> ("All Items List"=w1177:string[][])
        n719 = call <vilib>:"Acquire Semaphore.vi"("semaphore"=w1208) -> ("error out"=w1206:errorcluster, "semaphore out"=w1209:T13)  [unwired: 4 in, 1 out]
        n720 = Unbundle(w1211) -> ("counters 4ch"=w1199:T11)  [unwired: 1 out]
        "counters 4ch" <- w1199
        n721 = property on="path-file" class="Path"(error in=w1206) -> (error out=w1205:errorcluster, "Value"=w1204:path)  [unwired: 1 in, 1 out]
        n722 = call <instrlib>:"Counters4ch To Counters2ch.vi"("counters4ch"=w1199) -> ("counters2ch"=→"counters 2ch":T10)
        n723 = Array Subset "extract\nrecent data"(array=w1187, length=w1186) -> (w1185:T12)  [unwired: 1 in]
        n724 = call-poly <vilib>:"Write Delimited Spreadsheet.vi"("file path (dialog if empty)"=w1204, "2D data"=w1177, "append to file? (F)"=TRUE, "error in (no error)"=w1205, "delimiter (\\t)"=w1200) -> ("new file path (Not A Path if cancelled)"=w1203:path, "error out"=w1202:errorcluster)  [unwired: 9 in]
        n725 = property on="path-file" class="Path"(error in=w1202, "Value"=w1203) -> (error out=w1201:errorcluster)  [unwired: 1 in, 1 out]
        n726 = call <instrlib>:"data to graphs.vi"("data in"=w1185) -> ("graph coincidences"=→"graph coinc":cluster{timestamp[], u32[]}[], "graph singles"=w1192:cluster{timestamp[], u32[]}[])  [unwired: 9 in]
        n727 = call <vilib>:"Release Semaphore.vi"("error in (no error)"=w1201, "semaphore"=w1209) -> ()  [unwired: 4 in, 2 out]
        n728 = Index Array(array=w1192, index #1=0 ("index"), index #2=1 ("index"), index #3=2 ("index"), index #4=3 ("index")) -> (element #1=→"graph-A-S" →"graph-A":cluster{timestamp[], u32[]}, element #2=→"graph-B-S" →"graph-B":cluster{timestamp[], u32[]}, element #3=→"graph-C-S" →"graph-C":cluster{timestamp[], u32[]}, element #4=→"graph-D-S" →"graph-D":cluster{timestamp[], u32[]})
      }
      frame Error {
      }
    }
  }
  n729 = Unbundle(w6) -> ("semaphore files"=w28:T13, "semaphore port"=w27:T13, "notifier read request"=w22:refnum<notifier>, "queue data"=w25:refnum<queue>, "queue instructions"=w26:refnum<queue>)
  n730 = Release Queue(queue=w26, error in (no error)=w21) -> (error out=w43:errorcluster)  [unwired: 1 in, 2 out]
  n731 = Release Queue(queue=w25, error in (no error)=w43) -> (error out=w24:errorcluster)  [unwired: 1 in, 2 out]
  n732 = Release Notifier(notifier=w22, error in (no error)=w24) -> (error out=w23:errorcluster)  [unwired: 1 in, 2 out]
  n733 = call <vilib>:"Release Semaphore Reference.vi"("error in (no error)"=w23, "semaphore"=w27) -> ("error out"=w33:errorcluster)  [unwired: 8 in, 1 out]
  n734 = call <vilib>:"Release Semaphore Reference.vi"("error in (no error)"=w33, "semaphore"=w28) -> ("error out"=w10:errorcluster)  [unwired: 8 in, 1 out]
  n735 = disable-structure shown="RUN_TIME_ENGINE==True" {
    disable-tunnel: w10 -> [_ _]
    frame condition #0 (active) {
    }
    frame condition #1 {
      n736 = Quit LabVIEW() -> ()  [unwired: 1 in]
    }
  }
